vi "slow_control_2_07.vi"() -> ()   [LabVIEW 2018]
uses:
  <instrlib>/Lake Shore 335/Lake Shore 335.lvlib
  <instrlib>/CAEN PSM/CAEN PSM.lvlib
  <vilib>/DAQmx/read.llb/DAQmx Read (Analog 1D DBL NChan 1Samp).vi
  <resource>/objmgr/daqmx.rc
  ffb0d1b3-ef19-4e2e-b36e-7277177ef4b3.vi
  9a1acc8a-69db-4048-9e4c-bb07d66d2422.vi
  499f9cf5-7b15-41ea-951a-8da9be12721d.vi
  fa57f61f-0bb9-49ac-92eb-fcb40add4dbb.vi
  <vilib>/DAQmx/create/channels.llb/DAQmx Create Channel (AI-Temperature-RTD).vi
  <vilib>/DAQmx/create/channels.llb/DAQmx Create Channel (AI-Current-Basic).vi
  <vilib>/DAQmx/create/channels.llb/DAQmx Create Channel (AI-Voltage-Basic).vi
panel:
  out "Array 4":i32[](array[numeric])
  out "Array 3":i32[](array[numeric])
  out "Array 2":i32[](array[numeric])
  out "Timestamp last measured":timestamp
  out "Auto-clear":bool
  in  "Auto-clear data?":bool
  in  "Clear data":bool
  in  "Clear data every N cycles":dbl
  in  "N samples":i32=30
  out "Average Flow (SLPM)":dbl caption="Flow (SLPM)"
  out "Channel Names":string[](array[string])
  out "Heater":dbl
  out "Coldhead":dbl
  out "Cycle number":i32
  in  "Cycles to execute":dbl=5.0 format="%#_13g"
  out "Detector Pressure":dbl
  in  "N samples":i32=20
  in  "Allows tabs on \nfront panel":T1(tab)
  in  "Specify up to six temperature sensors inside \nthe detector, separated with a comma.\nNumbers only, single commas, no empty strings!":string="10,11,12,13,14,15"
  out "Valid example:":string="11,12, 13, 15 ,14 "
  in  "Anode ch.":enum16{"1", "2", "3", "4"}(ring)=enum."3"
  in  "CAEN unit selector":enum16{"CAEN 1", "CAEN 2"}(ring)
  in  "Multipliers":dbl[](array[numeric])=[1.0, 1.0, 1.0, 1.0, 1.0, 1.0, 1.0, 1.0]
  in  "Offsets\nsubtracted":dbl[](array[numeric])=[0.0, 0.0, 0.0, 0.0, 0.0, 0.0, 0.0, 0.0]
  in  "Channel Names (9207, ai8:15)":string[](array[string])=["i0", "i1", "i2", "i3", "i4", "i5", "i6", "i7"] caption="\"Other\""
  in  "Flow meter input:":T2(ring)=enum."v3"
  in  "Detector pressure input:":T2(ring)
  in  "Channel Names (9207, ai0:7)":string[](array[string])=["v0", "v1", "v2", "v3", "v4", "v5", "v6", "v7"] caption="\"Other\""
  in  "Multipliers":dbl[](array[numeric])=[0.2, 1.0, 1.0, 28.409091, 1.0, 1.0, 1.0, 1.0]
  in  "Offsets\nsubtracted":dbl[](array[numeric])=[0.002, 0.0, 0.0, 0.44376, 0.0, 0.0, 0.0, 0.0]
  in  "Voltage channels":tag[](array[tag])=["9207/ai0", "9207/ai1", "9207/ai2", "9207/ai3", "9207/ai4", "9207/ai5", "9207/ai6", "9207/ai7"]
  in  "COM-port CAEN 1":refnum<visa-resource-name>
  in  "COM-port CAEN 2":refnum<visa-resource-name>
  out "Temp B":dbl
  out "Temp A":dbl
  out "LakeShore readings 2":dbl[](array[numeric])
  in  "Run lakeshore?":bool
  in  "ID Query":bool=TRUE
  in  "COM-port LakeShore":refnum<visa-resource-name>
  in  "PID settings":cluster{"P":dbl, "I":dbl, "D":dbl}={"P"=50.0, "I"=20.0, "D"=120.0}
  in  "Setpoint (°C)":dbl=-100.0 format="%.1f"
  in  "Heater range":u16(ring) items=["Off", "Low (On)", "Medium", "High"]
  in  "Current channels":tag[](array[tag])=["9207/ai8", "9207/ai9", "9207/ai10", "9207/ai11", "9207/ai12", "9207/ai13", "9207/ai14", "9207/ai15"]
  in  "Channel Names (CAEN)":string[](array[string])=["PMT 1", "PMT 2", "Anode", "Cathode", "Top gate", "Bottom gate", "Other 1", "Other 2"]
  in  "RTD Type":i32(ring)=12481 items=["Pt3750"=12481, "Pt3851"=10071, "Pt3911"=12482, "Pt3916"=10069, "Pt3920"=10053, "Pt3928"=12483, "Custom"=10137]
  in  "Module 1 channels (slot 1)":tag[](array[tag])
  in  "Current Excitation Source":i32(ring)=10200 items=["Internal"=10200, "External"=10167, "None"=10230]
  in  "Resistance Configuration":i32(ring)=3 items=["2-Wire"=2, "3-Wire"=3, "4-Wire"=4]
  in  "R (T = 0°C):":dbl
  in  "B":dbl
  in  "A":dbl
  in  "C":dbl
  in  "Module 2 channels (slot 2)":tag[](array[tag])
  out "Det. T.":i32[](array[numeric])
  out "9207 (V; A) Converted":dbl[](array[numeric])
  out "9216 #1 (°C)":dbl[](array[numeric])
  out "9216 #2 (°C)":dbl[](array[numeric])
  out "Readouts (V, mA)":dbl[](array[numeric]) format="%0.2f"
  out "Det.P input #":i32
  out "Flow input #":i32
  in  "Repeat Alarm SMS\nevery N minutes":dbl=15.0
  in  "Test alarm":bool
  in  "Shut off heating if Alarm is active":bool
  out "Warning":bool
  in  "UPS":bool
  in  "UPS Voltage Threshold":dbl=220.0
  out "String 6":string
  out "String 5":string
  out "String 4":string
  out "String 3":string
  out "String 2":string
  out "String":string
  out "NI mod 2&3 status":bool
  in  "NI mod 2&3":bool
  in  "NI mod 1":bool
  in  "CAEN 2":bool
  in  "CAEN 1":bool
  in  "LakeShore":bool
  out "Det. P. warning":bool
  out "Boolean 6":bool
  out "Boolean 5":bool
  out "Boolean 4":bool
  out "Boolean 3":bool
  out "Boolean 2":bool
  out "Boolean":bool
  in  "T 6":bool
  in  "T 5":bool
  in  "T 4":bool
  in  "T 3":bool
  in  "T 2":bool
  in  "T 1":bool
  in  "Detector P":bool
  in  "Overpressure threshold":dbl
  in  "Underpressure threshold":dbl
  out "Comm. status":bool
  in  "High Temp threshold":dbl format="%#_13g"
  in  "Low Temp threshold":dbl format="%#_13g"
  in  "Ignore Initialization Errors":bool=TRUE caption="Ignore init. errors?"
  out "LakeShore status":bool
  out "NI mod1 (P) status":bool
  out "CAEN 1 status":bool
  out "CAEN 2 status":bool
  out "Initialization status":bool
  out "Minimum input voltage measured":dbl
  out "9207 (ai8:15, Amperes)":cluster{timestamp[], dbl[]}[](graph)
  in  "Temperature channel selector":u16(ring)=10 items=["11"=11, "12"=12, "13"=13, "14"=14, "15"=15, "16"=16, "17"=17, "Average"=666]
  out "Heater power (%)":cluster{timestamp[], dbl[]}[](graph)
  out "Flow (SLPM)":cluster{timestamp[], dbl[]}[](graph)
  out "9207 (ai0:7, Volts)":cluster{timestamp[], dbl[]}[](graph)
  out "Phase Diagram":cluster{"X":dbl, "Y":dbl}[](graph)
  out "Temperature":cluster{timestamp[], dbl[]}[](graph)
  in  "Pause?":bool
  out "Integrated Flow (SL)":dbl
  in  "Reset?":bool
  out "LakeShore readings":dbl[](array[numeric])
  in  "Temperature Channel Selector":u16(ring) items=["11"=11, "12"=12, "13"=13, "14"=14, "15"=15, "16"=16, "17"=17]
  out "Historical Large Phase Diagram":cluster{dbl[], dbl[]}[](graph)
  out "Large Phase Diagram":cluster{"X":dbl, "Y":dbl}[](graph)
  in  "Temperature Channel Selector":u16(ring)=666 items=["11"=11, "12"=12, "13"=13, "14"=14, "15"=15, "16"=16, "17"=17, "Average"=666]
  in  "Scale.Range:Minimum 8":dbl
  in  "Scale.Range:Maximum 8":dbl=4000.0
  in  "Scale.Range:Minimum 7":dbl
  in  "Scale.Range:Maximum 7":dbl=4000.0
  in  "Scale.Range:Minimum 6":dbl=-3000.0
  in  "Scale.Range:Maximum 6":dbl
  in  "Scale.Range:Minimum 5":dbl
  in  "Scale.Range:Maximum 5":dbl=3000.0
  in  "Scale.Range:Minimum 4":dbl=-5000.0
  in  "Scale.Range:Maximum 4":dbl
  in  "Scale.Range:Maximum 3":dbl=4000.0
  in  "Scale.Range:Minimum 3":dbl
  in  "Scale.Range:Maximum 2":dbl=1000.0
  in  "Scale.Range:Minimum 2":dbl
  out "CAEN 1.1":dbl(knob) scale=0.0..1000.0
  out "CAEN 1.1":string
  in  "Scale.Range:Maximum":dbl=1000.0
  in  "Scale.Range:Minimum":dbl
  out "CAEN 2.3 2":string
  out "CAEN 2.2 2":string
  out "Channel Names":string[](array[string])
  out "CAEN 2.3":dbl(knob) scale=0.0..4000.0
  out "CAEN 2.2":dbl(knob) scale=0.0..4000.0
  out "CAEN 2.1":string
  out "CAEN 2.0":string
  out "CAEN 1.3":string
  out "CAEN 1.2":string
  out "CAEN 1.0":string
  out "Channel Names":string[](array[string])
  in  "Set to zero":bool
  out "CAEN 2.1":dbl(knob)
  out "CAEN 2.0":dbl(knob) scale=0.0..3000.0
  in  "Apply Voltage":bool
  in  "VSet (V)":dbl[](array[numeric])
  in  "IMax (uA)":dbl[](array[numeric])
  in  "VMax (V)":dbl[](array[numeric])
  out "CAEN 1.3":dbl(knob)
  out "CAEN 1.2":dbl(knob) scale=0.0..4000.0
  out "CAEN 1.0":dbl(knob) scale=0.0..1000.0
  out "Vmon (V)":dbl[](array[numeric])
  out "IMon (uA)":dbl[](array[numeric])
  in  "Read V every N cycles":i16=120
  in  "Reset anode":bool
  in  "Kill every Y minutes":i32=10
  in  "Keep off for X seconds":i32=10
  out "?":bool
  out "Killed":bool
  out "Restarted":bool
  out "Anode times":dbl[](array[numeric]) format="%_12f"
  out "Anode times 2":timestamp[](array[timestamp])
  in  "Kill voltage":bool
  in  "stop":bool
  out "Voltages":dbl[](array[numeric])
  out "Started up?":bool
  out "TOBA appended":dbl[][](array[numeric])
  in  "Read T every N cycles":i32=2
  out "Time until next cycle":dbl format="%.3g"
  in  "Time per cycle (s)":i32=2 caption="Time Target (s)"
  # "<- Proof of concept for New/Old T + New P"
  # "Moving averages"
  # "NI 9216 Temperature settings"
  # "CAEN settings"
  # "NI 9207 Voltage settings"
  # "If RTD type is custom,\nspecify the Callendar-\nVan Dusen parameters"
  # "Anode connected to:"
  # "Channel:"
  # "Lakeshore settings"
  # "NI 9207 Current settings"
  # "Connection settings"
  # "Gain (P) (XX.X)"
  # "Reset (I) (XX.X)"
  # "Rate (D) (X.X%)"
  # "Move to Quick Temp tab ^"
  # "Thresholds"
  # "Alarm indicators and arms"
  # "Alarm conditions"
  # "Data"
  # "Time of last reset"
  # "Scale:"
  # "to"
  # "to"
  # "Scale:"
  # "Time of last reactivation"
  # "Settings"
  # "to"
  # "Scale:"
  # "to"
  # "Scale:"
  # "Scale:"
  # "to"
  # "Scale:"
  # "to"
  # "Scale:"
  # "to"
  # "to"
  # "Scale:"
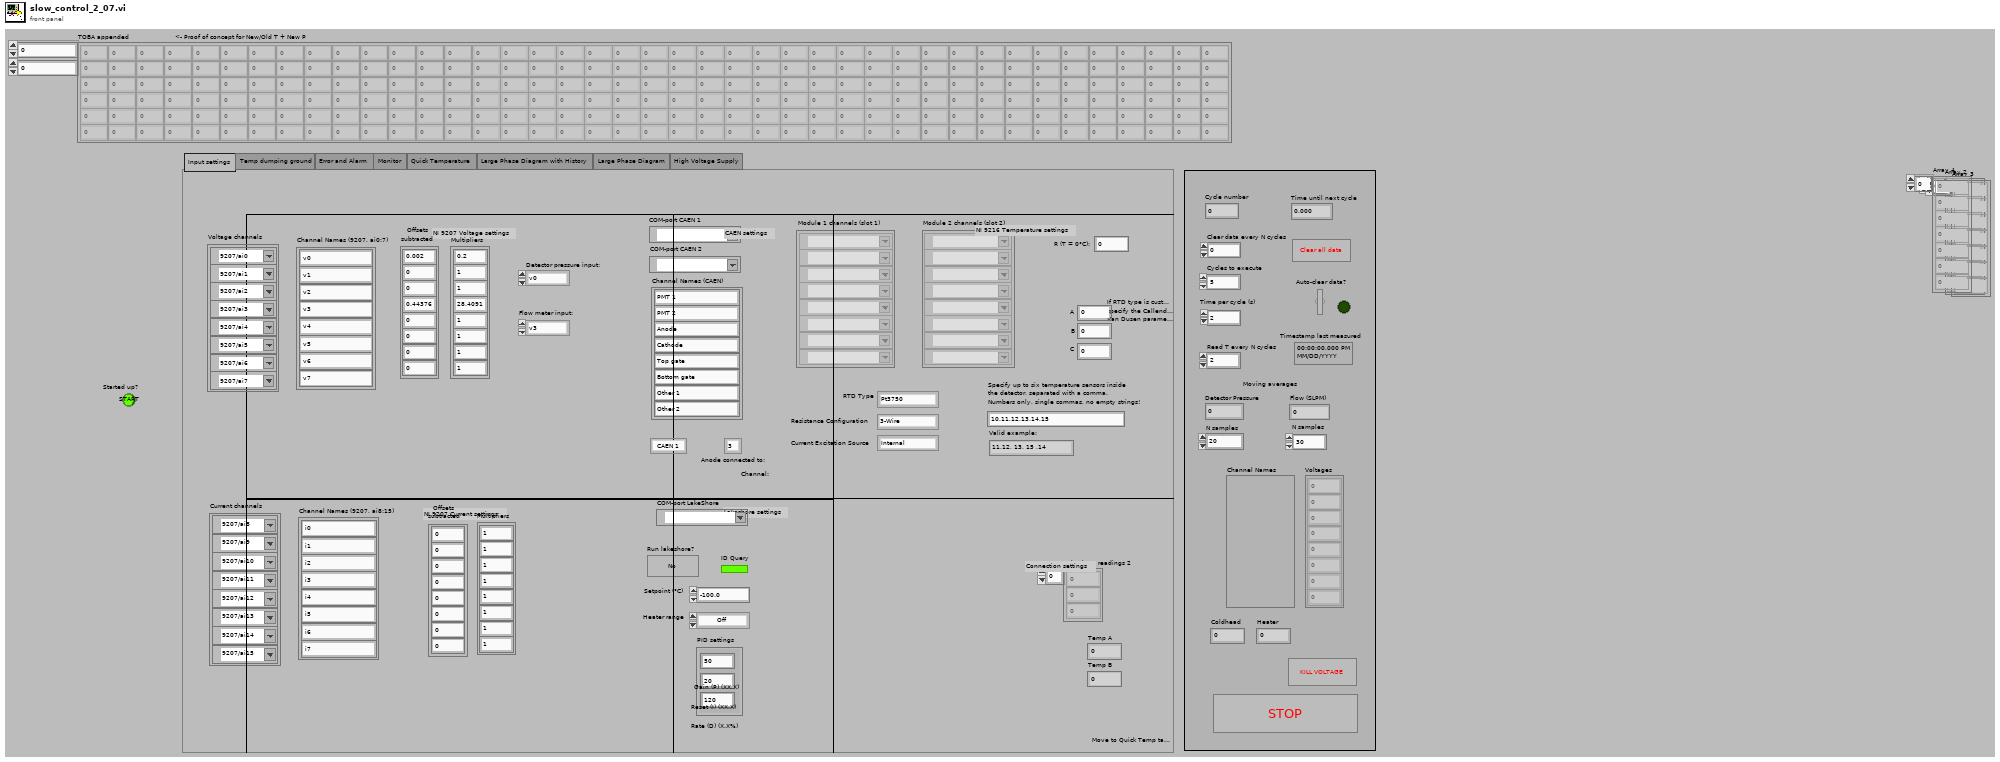
[diagram p1: front panel]
types:
  T1 = enum32{"Input settings", "Temp dumping ground", "Error and Alarm", "Monitor", "Quick Temperature", "Large Phase Diagram with History", "Large Phase Diagram", "High Voltage Supply"}
  T2 = enum16{"v0", "v1", "v2", "v3", "v4", "v5", "v6", "v7"}
  T3 = cluster{"Baud Rate":u32, "Parity":u16, "Data Bits":u16, "Stop Bits":u16, "Flow Control":u16}
  T4 = cluster{"VISA resource name out":refnum<visa-resource-name>, "error out":errorcluster}
  T5 = cluster{"task out":refnum<k21>, "error out":errorcluster}
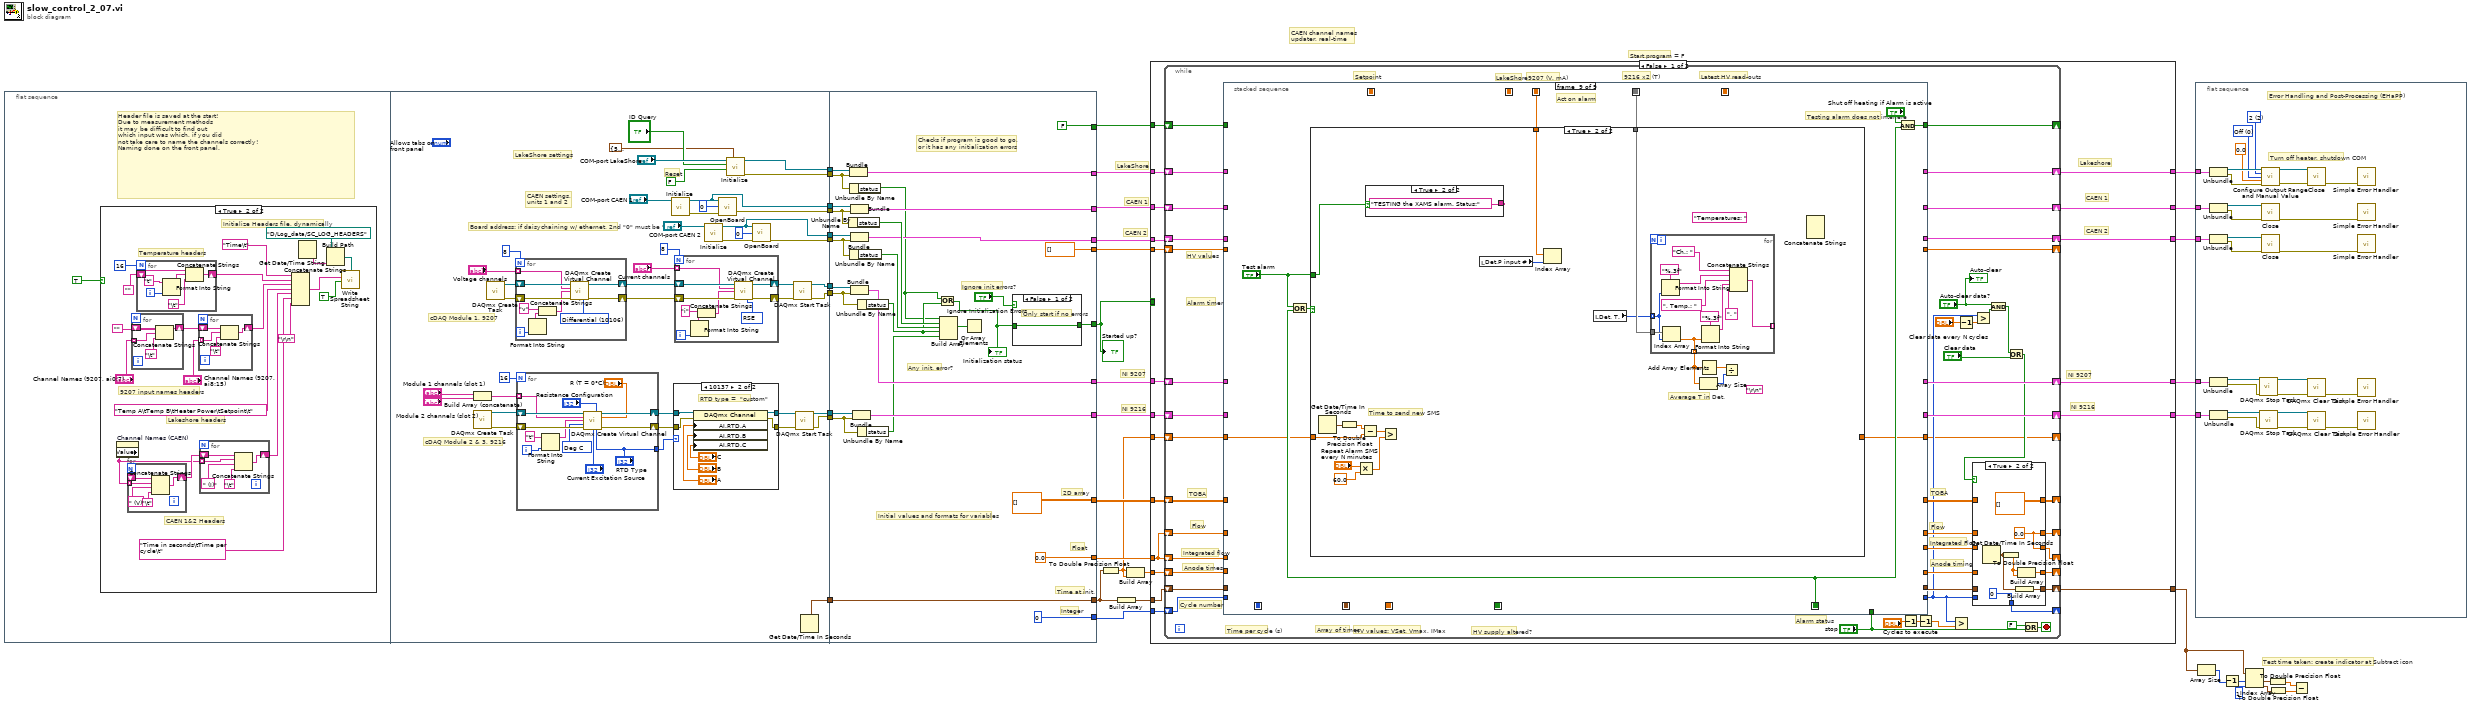
[diagram p0: block diagram]
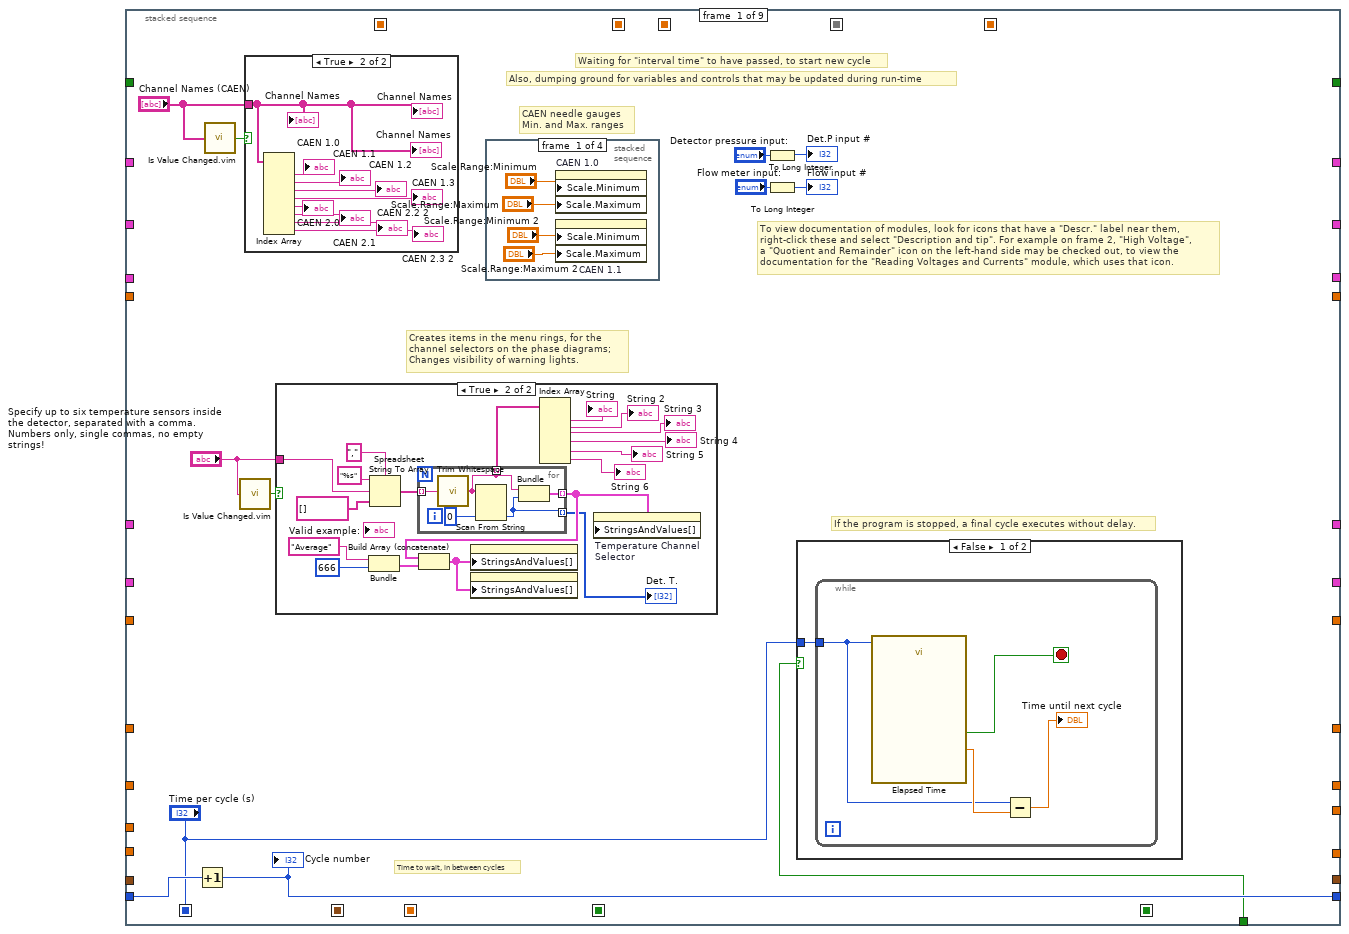
[diagram p3: hidden frame]
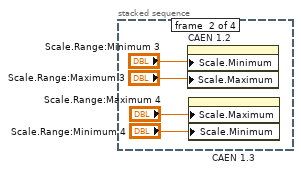
[diagram p6: hidden frame]
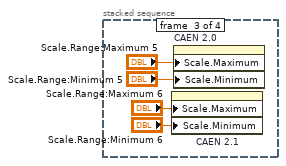
[diagram p7: hidden frame]
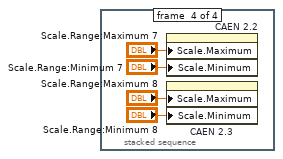
[diagram p8: hidden frame]
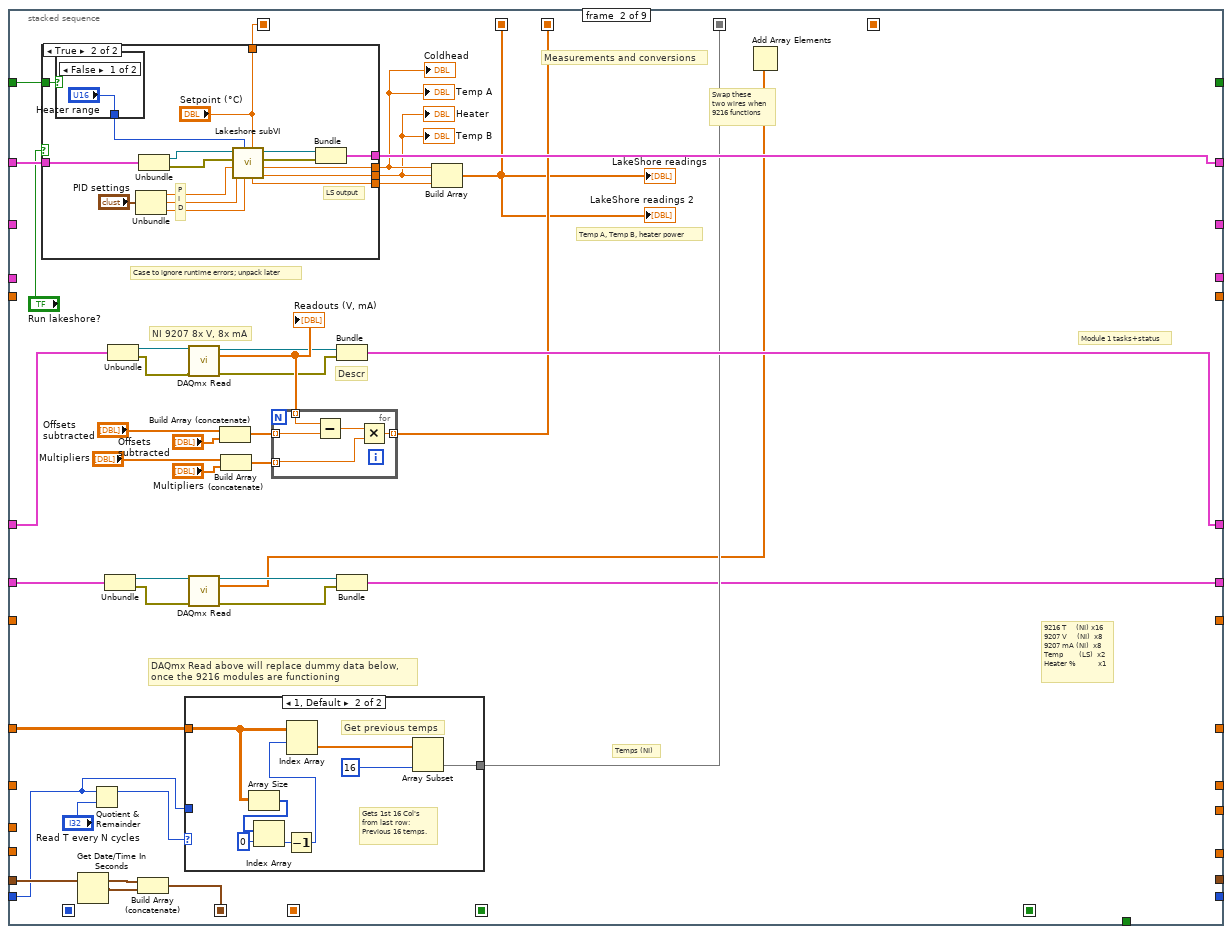
[diagram p10: hidden frame]
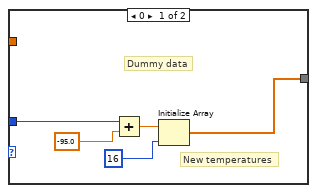
[diagram p11: hidden frame]
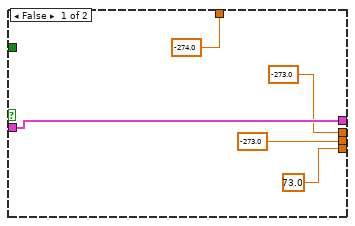
[diagram p12: hidden frame]
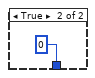
[diagram p13: hidden frame]
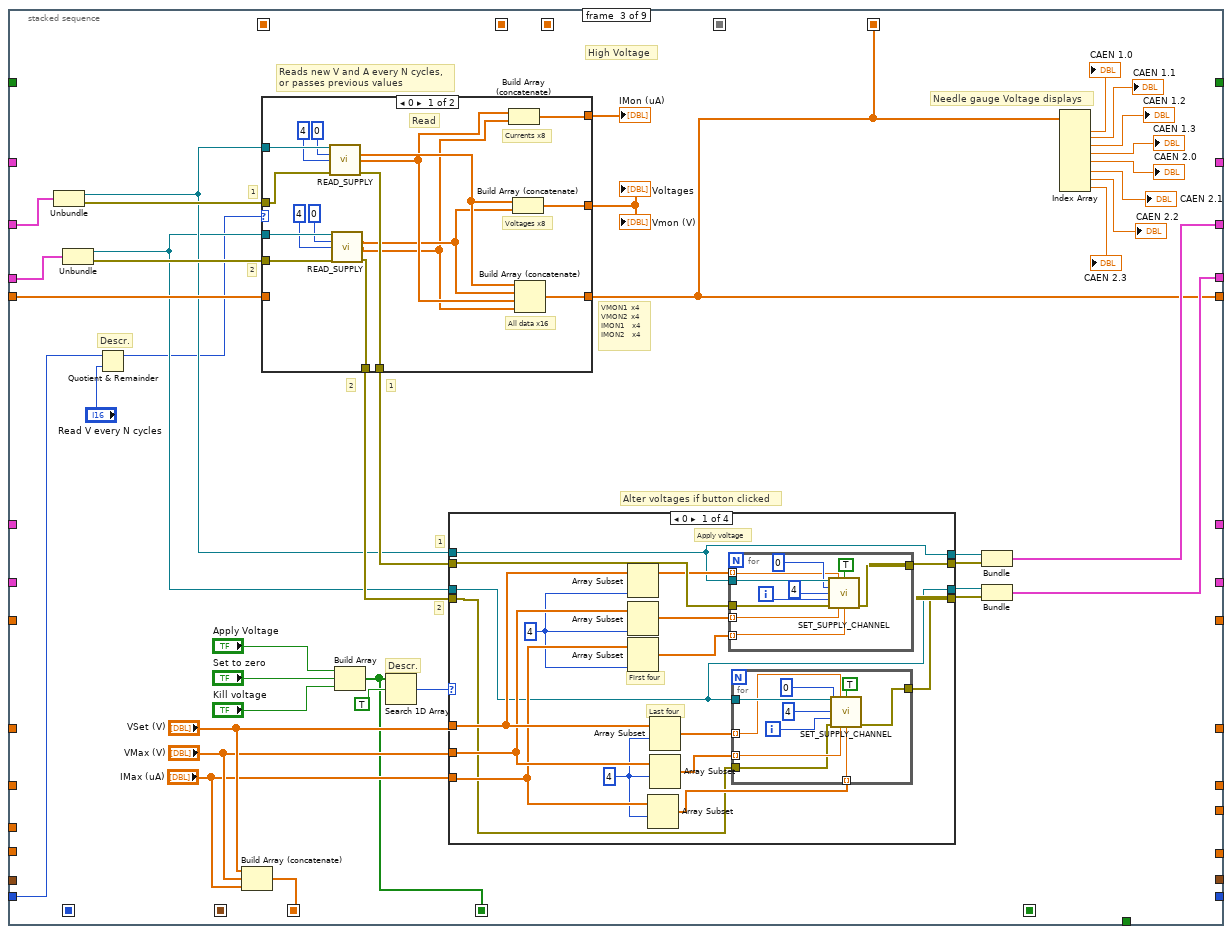
[diagram p14: hidden frame]
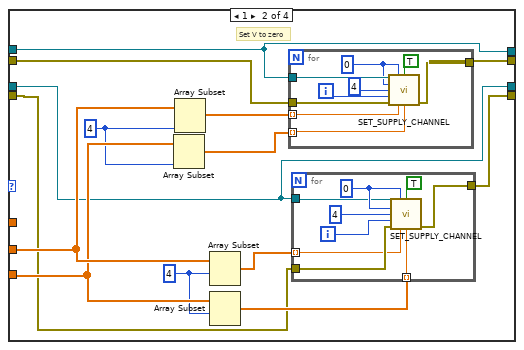
[diagram p15: hidden frame]
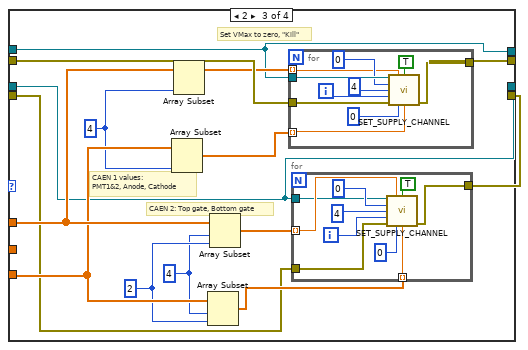
[diagram p16: hidden frame]
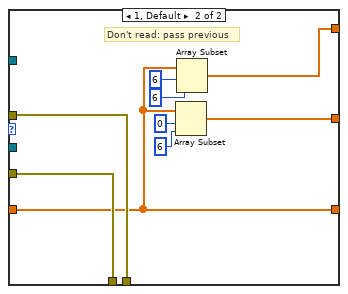
[diagram p18: hidden frame]
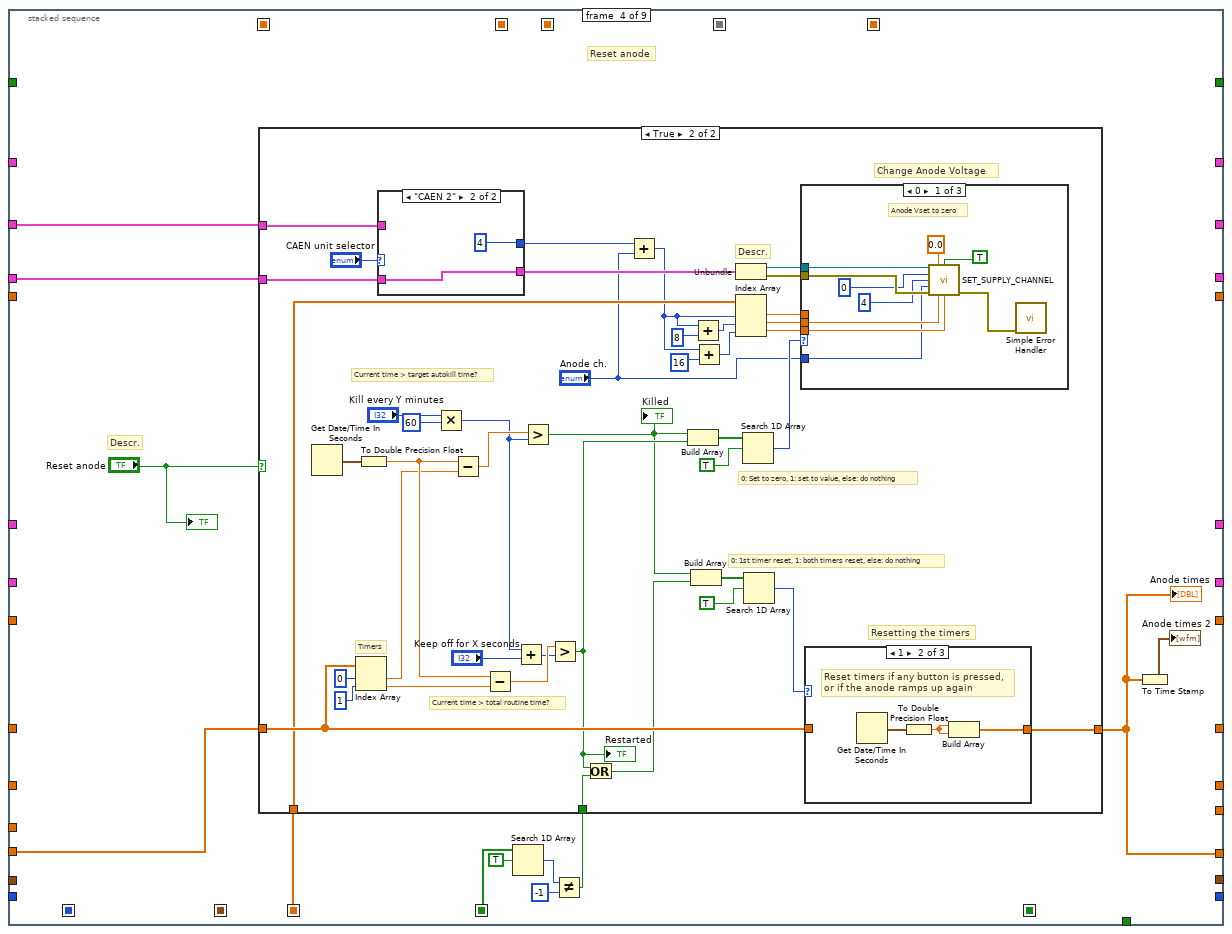
[diagram p19: hidden frame]
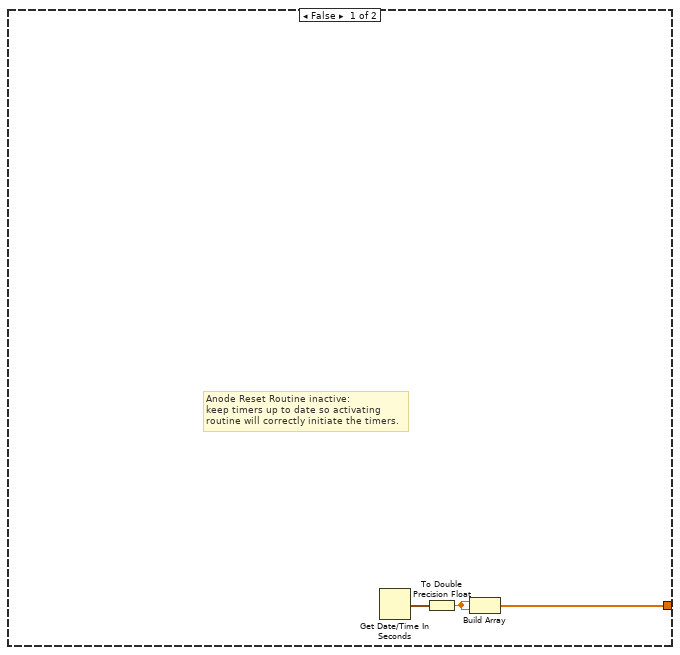
[diagram p20: hidden frame]
diagram:
  # "CAEN channel names\nupdater, real-time"
  # "NI 9216"
  # "Test time taken: create indicator at Subtract icon"
  # "NI 9207"
  # "Start program = F"
  # "CAEN 2"
  # "CAEN 1"
  # "LakeShore"
  n1 = flat-sequence {
    tunnel: [w123] -> w39
    tunnel: [w122] -> w38
    tunnel: [w110] -> w37
    tunnel: [w119] -> w36
    tunnel: [w100] -> w35
    tunnel: [w118] -> w30
    tunnel: [w114] -> w22
    tunnel: [w113] -> w21
    tunnel: [w101] -> w13
    tunnel: [w95] -> w5
    tunnel: [w94] -> w4
    tunnel: w39 -> [w195]
    tunnel: w38 -> [w194]
    tunnel: w37 -> [w192]
    tunnel: w36 -> [w191]
    tunnel: w35 -> [w181]
    tunnel: [w196] -> w19
    tunnel: [0.0] -> w18
    tunnel: [dbl[] []] -> w34
    tunnel: [dbl[][] []] -> w6
    tunnel: [0] -> w33
    tunnel: [w193] -> w32
    tunnel: [w190] -> w31
    tunnel: [w189] -> w17
    tunnel: w30 -> [w189]
    tunnel: w22 -> [w187]
    tunnel: w21 -> [w186]
    tunnel: [w185] -> w20
    tunnel: [FALSE] -> w14
    tunnel: w13 -> [w182]
    tunnel: [w180] -> w12
    tunnel: w5 -> [w172]
    tunnel: w4 -> [w171]
    tunnel: [w170] -> w3
    frame #0 {
      # "Header file is saved at the start!\nDue to measurement methods\nit may be difficult to find out\nwhich input was which, if you did\nnot take care to name the channels correctly!\nNaming done on the front panel."
      n2 = case shown="True" TRUE {
        frame False {
        }
        frame True {
          # "CAEN 1&2 Headers"
          # "Lakeshore headers"
          # "9207 input names headers"
          # "Temperature headers"
          # "Initialize Headers file, dynamically"
          n3 = property on="Channel Names (CAEN)" class="Arr (strict)"() -> ("Value"=w45:string[])  [unwired: 2 in, 2 out]
          n4 = for {
            tunnel: w45 -> [w69] mode=indexing
            shift-right: [w67] -> w46
            shift-left: _ -> [w66]
            n5 = Concatenate Strings(w66, w69, " (V)", "\t") -> (w67:string)
          }
          n6 = for {
            shift-right: [w77] -> w49
            shift-left: "" -> [w78]
            tunnel: "Channel Names (9207, ai0:7)" -> [w75] mode=indexing
            n7 = Concatenate Strings(w78, w75, "\t") -> (w77:string)
          }
          n8 = for {
            N: 16 -> [_]
            shift-right: [w79] -> w52
            shift-left: "" -> [w80]
            i -> [w84]
            n9 = Format Into String(initial string="t", w84) -> (resulting string=w82:string)  [unwired: 2 in, 1 out]
            n10 = Concatenate Strings(w80, w82, "\t") -> (w79:string)
          }
          n11 = for {
            shift-right: [w72] -> w48
            shift-left: w49 -> [w74]
            tunnel: "Channel Names (9207, ai8:15)" -> [w71] mode=indexing
            n12 = Concatenate Strings(w74, w71, "\t") -> (w72:string)
          }
          n13 = for {
            shift-right: [w62] -> w44
            shift-left: w46 -> [w63]
            tunnel: w45 -> [w61] mode=indexing
            n14 = Concatenate Strings(w63, w61, " (I)", "\t") -> (w62:string)
          }
          n15 = Concatenate Strings("Time\t", w52, w48, "Temp A\tTemp B\tHeater Power\tSetpoint\t", w44, "Time in seconds\tTime per cycle\t", "\r\n") -> (w51:string)
          n16 = Get Date/Time String() -> (date string=w55:string)  [unwired: 3 in, 1 out]
          n17 = Build Path(base path=path "D:/Log_data/SC_LOG_HEADERS" ("file path (dialog if empty)"), name or relative path=w55) -> (appended path=w56:path)
          n18 = call <vilib>:"Write Spreadsheet String.vi"("append to file? (new file:F)"=TRUE, "spreadsheet string"=w51, "file path (dialog if empty)"=w56) -> ()  [unwired: 7 in, 2 out]
        }
      }
    }
    frame #1 {
      # "cDAQ Module 2 & 3, 9216"
      # "cDAQ Module 1, 9207"
      # "Board address: if daisychaining w/ ethernet, 2nd \"0\" must be \"1\""
      # "CAEN settings,\nunits 1 and 2"
      # "Reset"
      # "LakeShore settings"
      n19 = call <vilib>:"DAQmx Create Task.vi"() -> ("task out"=w93:refnum<k21>, "error out"=w96:errorcluster)  [unwired: 14 in]
      n20 = Build Array (concatenate)("Module 1 channels (slot 1)", "Module 2 channels (slot 2)") -> (w90:tag[])
      n21 = call <vilib>:"DAQmx Create Task.vi"() -> ("task out"=w109:refnum<k21>, "error out"=w108:errorcluster)  [unwired: 14 in]
      n22 = for {
        N: 8 -> [_]
        shift-right: [w164] -> w105
        shift-left: w109 -> [w163]
        shift-right: [w165] -> w104
        shift-left: w108 -> [w161]
        tunnel: "Voltage channels" -> [w162] mode=indexing
        i -> [w167]
        w159 = 10106 items=["Default"=-1, "RSE"=10083, "NRSE"=10078, "Differential"=10106, "Pseudodifferential"=12529] ("input terminal configuration")
        n23 = Format Into String(w167) -> (resulting string=w166:string)  [unwired: 3 in, 1 out]
        n24 = Concatenate Strings("v" ("string"), w166) -> (w160:string)
        n25 = call-poly <vilib>:"DAQmx Create Virtual Channel.vi"("task in"=w163, "input terminal configuration"=w159, "physical channels"=w162, "name to assign"=w160, "error in"=w161) -> ("task out"=w164:refnum<k21>, "error out"=w165:errorcluster)  [unwired: 9 in]
      }
      n26 = for {
        N: 16 -> [_]
        shift-right: [w145] -> w89
        shift-left: w93 -> [w148]
        shift-right: [w146] -> w88
        shift-left: w96 -> [w147]
        tunnel: w90 -> [w144] mode=indexing
        tunnel: ["RTD Type"] -> w85
        i -> [w142]
        w139 = 10143 items=["Deg C"=10143, "Deg F"=10144, "Kelvins"=10325, "Deg R"=10145, "From Custom Scale"=10065] ("units")
        n27 = Format Into String(initial string="t", w142) -> (resulting string=w141:string)  [unwired: 2 in, 1 out]
        n28 = call-poly <vilib>:"DAQmx Create Virtual Channel.vi"("task in"=w148, "resistance configuration"="Resistance Configuration", "physical channels"=w144, "r0"="R (T = 0°C):", "name to assign"=w141, "units"=w139, "error in"=w147, "current excitation source"="Current Excitation Source", "rtd type"="RTD Type") -> ("task out"=w145:refnum<k21>, "error out"=w146:errorcluster)  [unwired: 5 in]
      }
      n29 = call <instrlib>:"Initialize.vi"("VISA resource name"="COM-port CAEN 1") -> ("error out"=w120:errorcluster, "VISA resource name out"=w110:refnum<visa-resource-name>)  [unwired: 9 in]
      n30 = case shown="10137" w85 {
        tunnel: w89 -> [w128 w132]
        tunnel: w88 -> [w127 w131]
        tunnel: [w128 w130] -> w87
        tunnel: [w127 w129] -> w86
        frame 0, Default {
          # "Don't need to specify the A, B, C\nvalues if RTD type is not \"custom\""
        }
        frame 10137 {
          # "RTD type =  \"custom\""
          n31 = property class="DAQmx Channel"(reference=w132, error in=w131, "AI.RTD.A"="A", "AI.RTD.B"="B", "AI.RTD.C"="C") -> (reference out=w130:refnum<k21>, error out=w129:errorcluster)
        }
      }
      n32 = for {
        N: 8 -> [_]
        shift-right: [w150] -> w102
        shift-left: w105 -> [w157]
        shift-right: [w149] -> w103
        shift-left: w104 -> [w156]
        tunnel: "Current channels" -> [w155] mode=indexing
        i -> [w154]
        w158 = 10083 items=["default"=-1, "RSE"=10083, "NRSE"=10078, "Differential"=10106, "Pseudodifferential"=12529] ("input terminal configuration")
        n33 = Format Into String(w154) -> (resulting string=w152:string)  [unwired: 3 in, 1 out]
        n34 = Concatenate Strings("i", w152) -> (w151:string)
        n35 = call-poly <vilib>:"DAQmx Create Virtual Channel.vi"("task in"=w157, "input terminal configuration"=w158, "physical channels"=w155, "name to assign"=w151, "error in"=w156) -> ("task out"=w150:refnum<k21>, "error out"=w149:errorcluster)  [unwired: 9 in]
      }
      n36 = call <instrlib>:"Initialize.vi"("VISA resource name"="COM-port CAEN 2") -> ("error out"=w115:errorcluster, "VISA resource name out"=w114:refnum<visa-resource-name>)  [unwired: 9 in]
      n37 = call <instrlib>:"OpenBoard.vi"("error in (no error)"=w120, "Board Address"=0, "VISA resource name"=w110) -> ("error out"=w119:errorcluster)  [unwired: 7 in, 1 out]
      n38 = call <instrlib>:"Initialize.vi"("Serial Configuration"=T3 {"Baud Rate"=57600, "Parity"=1, "Data Bits"=7, "Stop Bits"=10, "Flow Control"=0}, "Reset (True)"=FALSE ("Reset (LakeShore)"), "ID Query (True)"="ID Query", "VISA resource name"="COM-port LakeShore") -> ("error out"=w122:errorcluster, "VISA resource name out"=w123:refnum<visa-resource-name>)  [unwired: 6 in]
      n39 = call <instrlib>:"OpenBoard.vi"("error in (no error)"=w115, "Board Address"=u8 0, "VISA resource name"=w114) -> ("error out"=w113:errorcluster)  [unwired: 7 in, 1 out]
      n40 = call <vilib>:"DAQmx Start Task.vi"("task/channels in"=w102, "error in"=w103) -> ("task out"=w101:refnum<k21>, "error out"=w100:errorcluster)  [unwired: 12 in]
      n41 = call <vilib>:"DAQmx Start Task.vi"("task/channels in"=w87, "error in"=w86) -> ("task out"=w95:refnum<k21>, "error out"=w94:errorcluster)  [unwired: 12 in]
      n42 = Get Date/Time In Seconds() -> (seconds since 1Jan1904=w118:timestamp)
    }
    frame #2 {
      # "Initial values and formats for variables"
      # "Time at init."
      # "Integer"
      # "2D array"
      # "Float"
      # "Checks if program is good to go,\nor it has any initialization errors"
      # "Ignore init errors?"
      # "Any init. error?"
      n43 = Unbundle By Name(w191) -> ("status"=w197:bool)
      n44 = Unbundle By Name(w194) -> ("status"=w174:bool)
      n45 = Bundle("VISA resource name out"=w195, "error out"=w194) -> (w193:T4)  [unwired: 1 in]
      n46 = Unbundle By Name(w186) -> ("status"=w188:bool)
      n47 = Bundle("VISA resource name out"=w187, "error out"=w186) -> (w185:T4)  [unwired: 1 in]
      n48 = Bundle("task out"=w182, "error out"=w181) -> (w180:T5)  [unwired: 1 in]
      n49 = Bundle("VISA resource name out"=w192, "error out"=w191) -> (w190:T4)  [unwired: 1 in]
      n50 = Bundle("task out"=w172, "error out"=w171) -> (w170:T5)  [unwired: 1 in]
      n51 = Unbundle By Name(w181) -> ("status"=w175:bool)
      n52 = Unbundle By Name(w171) -> ("status"=w169:bool)
      n53 = Or(x=w174, y=w175) -> (x .or. y?=w173:bool)
      "Initialization status" <- w173
      n54 = Build Array(w174, w197, w175, w188, w169) -> (w198:bool[])
      n55 = Or Array Elements(Boolean array=w198) -> ()  [unwired: 1 out]
      n56 = case shown="False" "Ignore Initialization Errors" {
        tunnel: [w199 FALSE] -> w196
        tunnel: w173 -> [w199 _]
        frame False {
          # "Only start if no errors"
        }
        frame True {
          # "Always start program"
        }
      }
    }
  }
  n57 = To Double Precision Float(number=w17) -> (double precision float=w1:dbl)
  n58 = Build Array(w17) -> (w29:timestamp[])
  n59 = Build Array(w1, w1) -> (w16:dbl[])
  n60 = case shown="False" w19 {
    selector: w19 -> [_ w951]
    tunnel: [_ w951] -> _
    tunnel: w34 -> [w212 _]
    tunnel: w33 -> [w219 _]
    tunnel: w6 -> [w218 _]
    tunnel: w32 -> [w213 w949]
    tunnel: w31 -> [w215 w948]
    tunnel: w29 -> [w217 _]
    tunnel: [w216 timestamp[] []] -> w25
    tunnel: w20 -> [w214 w947]
    tunnel: w18 -> [w208 _]
    tunnel: w16 -> [w211 _]
    tunnel: [w210 w949] -> w15
    tunnel: w14 -> [w209 _]
    tunnel: w12 -> [w207 w946]
    tunnel: [w206 w948] -> w11
    tunnel: [w205 w947] -> w10
    tunnel: [w204 w946] -> w9
    tunnel: w3 -> [w203 w945]
    tunnel: [w202 w945] -> w2
    tunnel: w1 -> [w201 _]
    frame False {
      # "NI 9216"
      # "NI 9207"
      # "CAEN 2"
      # "CAEN 1"
      # "Lakeshore"
      n61 = while {
        shift-right: [w228] -> _
        shift-left: w219 -> [w266]
        shift-right: [w241] -> _
        shift-left: w218 -> [w255]
        shift-right: [w233] -> w216
        shift-left: w217 -> [w263]
        shift-right: [w257] -> w206
        shift-left: w215 -> [w250]
        shift-right: [w259] -> _
        shift-left: w212 -> [w262]
        shift-right: [w256] -> w205
        shift-left: w214 -> [w261]
        shift-right: [w258] -> w210
        shift-left: w213 -> [w260]
        shift-right: [w237] -> _
        shift-left: w208 -> [w252]
        shift-right: [w239] -> _
        shift-left: w208 -> [w253]
        shift-right: [w235] -> _
        shift-left: w211 -> [w251]
        shift-right: [w222] -> _
        shift-left: w209 -> [w249]
        shift-right: [w247] -> w204
        shift-left: w207 -> [w248]
        shift-right: [w245] -> w202
        shift-left: w203 -> [w246]
        shift-right: [w220] -> _
        shift-left: w201 -> [w221]
        stop <- w264 stop-if-true
        # "Alarm timer"
        # "Alarm status"
        # "LakeShore"
        # "9216 x2 (T)"
        # "9207 (V, mA)"
        # "HV supply altered?"
        # "Setpoint"
        # "Anode timing"
        # "Anode times"
        # "Integrated flow"
        # "Flow"
        # "Flow"
        # "Integrated Flow"
        # "TOBA"
        # "Array of times"
        # "Latest HV read-outs"
        # "Time per cycle (s)"
        # "Cycle number"
        # "HV values: VSet, Vmax, IMax"
        # "HV values"
        # "TOBA"
        n62 = stacked-sequence {
          seq-local: [_ _ w433 _ _ _ _ _ _] -> [_ _ _ w605 _ _ _ _ _]
          seq-local: ["Time per cycle (s)" _ _ _ _ _ _ _ _] -> [_ _ _ _ _ _ w814 _ _]
          seq-local: [_ _ w424 _ _ _ _ _ _] -> [_ _ _ _ _ _ w816 _ _]
          seq-local: [_ w377 _ _ _ _ _ _ _] -> [_ _ _ _ w696 w716 _ _ _]
          seq-local: [_ _ w427 _ _ _ _ _ _] -> [_ _ _ w608 _ _ _ _ _]
          seq-local: [_ w370 _ _ _ _ _ _ _] -> [_ _ _ _ _ _ w831 _ _]
          seq-local: [_ w365 _ _ _ _ _ _ _] -> [_ _ _ _ w691 w741 w818 w873 w910]
          seq-local: [_ w364 _ _ _ _ _ _ _] -> [_ _ _ _ w690 w732 w819 w877 w909]
          seq-local: [_ w352 _ _ _ _ _ _ _] -> [_ _ _ _ w689 w739 w817 _ _]
          seq-local: [_ _ _ _ _ _ _ w833 _] -> [_ _ _ _ _ _ _ _ w912]
          tunnel: [w290 _ _ _ _ _ _ _ _] -> w227
          tunnel: "stop" -> [w289 _ _ _ _ _ _ _ _]
          tunnel: w266 -> [w291 w366 w455 _ _ _ _ _ _]
          tunnel: w255 -> [_ w367 _ _ _ w742 _ _ _]
          tunnel: [_ _ _ _ _ w718 _ _ _] -> w242
          tunnel: w263 -> [_ w379 _ _ _ _ _ _ _]
          tunnel: w250 -> [_ _ w462 w606 _ _ _ w893 _]
          tunnel: w262 -> [_ _ w460 _ _ _ _ _ _]
          tunnel: w261 -> [_ _ w459 w597 _ _ _ w892 _]
          tunnel: w260 -> [_ w380 _ _ _ _ _ w891 _]
          tunnel: [_ w381 _ _ _ _ _ _ _] -> w258
          tunnel: [_ _ w424 _ _ _ _ _ _] -> w259
          tunnel: [_ _ w441 _ _ _ _ _ _] -> w257
          tunnel: [_ _ w438 _ _ _ _ _ _] -> w256
          tunnel: [_ _ _ _ _ w716 _ _ _] -> w234
          tunnel: w252 -> [_ _ _ _ w694 _ _ _ _]
          tunnel: w253 -> [_ _ _ _ w695 _ _ _ _]
          tunnel: w251 -> [_ _ _ w607 _ _ _ _ _]
          tunnel: [_ _ _ w601 _ _ _ _ _] -> w236
          tunnel: w249 -> [_ w373 _ _ _ _ _ _ _]
          tunnel: w248 -> [_ w372 _ _ _ _ _ w890 _]
          tunnel: [_ w368 _ _ _ _ _ _ _] -> w247
          tunnel: [_ _ _ _ w693 _ _ _ _] -> w238
          tunnel: [_ _ _ _ w692 _ _ _ _] -> w240
          tunnel: w246 -> [_ w351 _ _ _ _ _ w878 _]
          tunnel: [_ w346 _ _ _ _ _ _ _] -> w245
          tunnel: [_ _ _ _ _ _ _ _ w914] -> w222
          tunnel: w221 -> [_ _ _ _ _ _ _ _ w908]
          tunnel: [_ _ _ _ _ _ _ _ w907] -> w220
          frame #0 {
            # "Creates items in the menu rings, for the channel selectors on the phase diagrams;\nChanges visibility of warning lights."
            # "Also, dumping ground for variables and controls that may be updated during run-time"
            # "CAEN needle gauges\nMin. and Max. ranges"
            # "To view documentation of modules, look for icons that have a \"Descr.\" label near them,\nright-click these and select \"Description and tip\". For example on frame 2, \"High Voltage\",\na \"Quotient and Remainder\" icon on the left-hand side may be checked out, to view the\ndocumentation for the \"Reading Voltages and Currents\" module, which uses that icon."
            # "Time to wait, in between cycles"
            # "If the program is stopped, a final cycle executes without delay."
            # "Waiting for \"interval time\" to have passed, to start new cycle"
            n63 = Increment(x=w291) -> (x+1=w290:i32)
            "Cycle number" <- w290
            n64 = call "Is Value Changed.vim"("value"="Channel Names (CAEN)") -> ("changed or first call?"=w280:bool)
            n65 = call "Is Value Changed.vim"("value"="Specify up to six temperature sensors inside \nthe detector, separated with a comma.\nNumbers only, single commas, no empty strings!") -> ("changed or first call?"=w282:bool)
            n66 = case shown="True" w280 {
              tunnel: "Channel Names (CAEN)" -> [_ w292]
              frame False {
              }
              frame True {
                n67 = Index Array(array=w292) -> (element #1=→"CAEN 1.0":string, element #2=→"CAEN 1.1":string, element #3=→"CAEN 1.2":string, element #4=→"CAEN 1.3":string, element #5=→"CAEN 2.0":string, element #6=→"CAEN 2.1":string, element #7=→"CAEN 2.2 2":string, element #8=→"CAEN 2.3 2":string)  [unwired: 8 in]
                "Channel Names" <- w292
                "Channel Names" <- w292
                "Channel Names" <- w292
              }
            }
            n68 = case shown="True" w282 {
              tunnel: "Specify up to six temperature sensors inside \nthe detector, separated with a comma.\nNumbers only, single commas, no empty strings!" -> [_ w302]
              frame False {
              }
              frame True {
                n69 = Bundle("Average", 666) -> (w308:cluster{string, i32})  [unwired: 1 in]
                n70 = Spreadsheet String To Array(delimiter (Tab)=",", format string="%s", spreadsheet string=w302, array type (2D Dbl)=string[] []) -> (array=w311:string[])
                n71 = for {
                  tunnel: w311 -> [w323] mode=indexing
                  tunnel: [w321] -> w310 mode=indexing
                  tunnel: [w320] -> w301 mode=indexing
                  tunnel: [w319] -> w312 mode=indexing
                  n72 = call <vilib>:"Trim Whitespace.vi"("string"=w323) -> ("trimmed string"=w319:string)  [unwired: 1 in]
                  n73 = Scan From String(input string=w319, default 1=0) -> (output 1=w320:i32)  [unwired: 3 in, 3 out]
                  n74 = Bundle("trimmed string"=w319, w320) -> (w321:cluster{"trimmed string":string, i32})  [unwired: 1 in]
                }
                "Det. T." <- w301
                n75 = Build Array (concatenate)(w310, w308) -> (w309:cluster{"trimmed string":string, i32}[])
                n76 = property on="Temperature channel selector" class="Ring (strict)"("StringsAndValues[]"=w309) -> ()  [unwired: 2 in, 2 out]
                n77 = property on="Temperature Channel Selector" class="Ring (strict)"("StringsAndValues[]"=w309) -> ()  [unwired: 2 in, 2 out]
                n78 = Index Array(array=w312) -> (element #1=→"String":string, element #2=→"String 2":string, element #3=→"String 3":string, element #4=→"String 4":string, element #5=→"String 5":string, element #6=→"String 6":string)  [unwired: 6 in]
                n79 = property on="Temperature Channel Selector" class="Ring (strict)"("StringsAndValues[]"=w310) -> ()  [unwired: 2 in, 2 out]
              }
            }
            n80 = stacked-sequence {
              frame #0 {
                n81 = property on="CAEN 1.0" class="Knob (strict)"("Scale.Minimum"="Scale.Range:Minimum", "Scale.Maximum"="Scale.Range:Maximum") -> ()  [unwired: 2 in, 2 out]
                n82 = property on="CAEN 1.1" class="Knob (strict)"("Scale.Minimum"="Scale.Range:Minimum 2", "Scale.Maximum"="Scale.Range:Maximum 2") -> ()  [unwired: 2 in, 2 out]
              }
              frame #1 {
                n83 = property on="CAEN 1.2" class="Knob (strict)"("Scale.Minimum"="Scale.Range:Minimum 3", "Scale.Maximum"="Scale.Range:Maximum 3") -> ()  [unwired: 2 in, 2 out]
                n84 = property on="CAEN 1.3" class="Knob (strict)"("Scale.Maximum"="Scale.Range:Maximum 4", "Scale.Minimum"="Scale.Range:Minimum 4") -> ()  [unwired: 2 in, 2 out]
              }
              frame #2 {
                n85 = property on="CAEN 2.1" class="Knob (strict)"("Scale.Maximum"="Scale.Range:Maximum 6", "Scale.Minimum"="Scale.Range:Minimum 6") -> ()  [unwired: 2 in, 2 out]
                n86 = property on="CAEN 2.0" class="Knob (strict)"("Scale.Maximum"="Scale.Range:Maximum 5", "Scale.Minimum"="Scale.Range:Minimum 5") -> ()  [unwired: 2 in, 2 out]
              }
              frame #3 {
                n87 = property on="CAEN 2.2" class="Knob (strict)"("Scale.Maximum"="Scale.Range:Maximum 7", "Scale.Minimum"="Scale.Range:Minimum 7") -> ()  [unwired: 2 in, 2 out]
                n88 = property on="CAEN 2.3" class="Knob (strict)"("Scale.Maximum"="Scale.Range:Maximum 8", "Scale.Minimum"="Scale.Range:Minimum 8") -> ()  [unwired: 2 in, 2 out]
              }
            }
            n89 = To Long Integer(number="Detector pressure input:") -> (32bit integer=→"Det.P input #":i32)
            n90 = To Long Integer(number="Flow meter input:") -> (32bit integer=→"Flow input #":i32)
            n91 = case shown="False" w289 {
              tunnel: "Time per cycle (s)" -> [w340 _]
              frame False {
                n92 = while {
                  tunnel: w340 -> [w342]
                  stop <- w344 stop-if-true
                  n93 = call "Elapsed Time"("Time Target (s)"=w342) -> ("Elapsed Time (s)"=w343:dbl, "Time has Elapsed"=w344:bool)  [unwired: 11 in, 6 out]
                  n94 = Subtract(x=w342, y=w343) -> (x-y=→"Time until next cycle":dbl)
                }
              }
              frame True {
              }
            }
          }
          frame #1 {
            # "DAQmx Read above will replace dummy data below,\nonce the 9216 modules are functioning"
            # "Swap these\ntwo wires when\n9216 functions"
            # "Descr"
            # "NI 9207 8x V, 8x mA"
            # "Case to ignore runtime errors; unpack later"
            # "Module 1 tasks+status"
            # "Temps (NI)"
            # "9216 T     (NI) x16\n9207 V     (NI)  x8\n9207 mA (NI)  x8\nTemp        (LS)  x2\nHeater %           x1"
            # "Temp A, Temp B, heater power"
            # "Measurements and conversions"
            n95 = case shown="True" "Run lakeshore?" {
              tunnel: [w404 w412] -> w381
              tunnel: w380 -> [w404 w411]
              tunnel: [-273.0 ("Input A") w410] -> w376
              tunnel: [-273.0 ("Input B") w409] -> w375
              tunnel: [73.0 ("Heater 1 (%)") w408] -> w374
              tunnel: w373 -> [_ w407]
              tunnel: [-274.0 "Setpoint (°C)"] -> w370
              frame False {
              }
              frame True {
                # "LS output"
                # "P\nI\nD"
                n96 = case shown="False" w407 {
                  tunnel: ["Heater range" 0] -> w415
                  frame False {
                  }
                  frame True {
                  }
                }
                n97 = Unbundle("PID settings") -> ("P"=w418:dbl, "I"=w417:dbl, "D"=w416:dbl)
                n98 = Unbundle(w411) -> ("VISA resource name out"=w420:refnum<visa-resource-name>, "error out"=w419:errorcluster)
                n99 = call "Lakeshore subVI.vi"("Setpoint"="Setpoint (°C)", "Rate (D) (X.X %)"=w416, "Range"=w415, "Reset (I) (XX.X)"=w417, "Gain (P) (XX.X)"=w418, "error in (no error)"=w419, "VISA resource name"=w420) -> ("Input B"=w409:dbl, "Input A"=w410:dbl, "error out"=w413:errorcluster, "VISA resource name out"=w414:refnum<visa-resource-name>, "Heater 1 (%)"=w408:dbl)
                n100 = Bundle("VISA resource name out"=w414, "error out"=w413) -> (w412:T4)  [unwired: 1 in]
              }
            }
            "Temp A" <- w376
            "Temp B" <- w375
            "Heater" <- w375
            "Coldhead" <- w376
            n101 = Get Date/Time In Seconds() -> (seconds since 1Jan1904=w378:timestamp)
            n102 = Quotient & Remainder(x=w366, y="Read T every N cycles") -> (x-y*floor(x/y)=w369:i32)  [unwired: 1 out]
            n103 = Unbundle(w351) -> ("task out"=w350:refnum<k21>, "error out"=w349:errorcluster)
            n104 = Unbundle(w372) -> ("task out"=w356:refnum<k21>, "error out"=w355:errorcluster)
            n105 = Build Array (concatenate)(w379, w378) -> (w377:timestamp[])
            n106 = case shown="1, Default" w369 {
              tunnel: w367 -> [_ w397]
              tunnel: [w390 w393] -> w364
              tunnel: w366 -> [w389 _]
              frame 0 {
                # "Dummy data"
                # "New temperatures"
                n107 = Add(x=w389, y=-95.0 ("element")) -> (x+y=w392:dbl)
                n108 = Initialize Array(w392, 16) -> (w390:dbl[])
              }
              frame 1, Default {
                # "Gets 1st 16 Col's\nfrom last row:\nPrevious 16 temps."
                # "Get previous temps"
                n109 = Array Size(array=w397) -> (size(s)=w399:i32[])
                n110 = Index Array(array=w399, index=0) -> (element=w400:i32)
                n111 = Decrement(x=w400) -> (x-1=w396:i32)
                n112 = Index Array(array=w397, index (row)=w396) -> (element=w395:dbl[])  [unwired: 1 in]
                n113 = Array Subset(array=w395, length=16) -> (w393:dbl[])  [unwired: 1 in]
              }
            }
            n114 = call-poly <vilib>:"DAQmx Read.vi"("task/channels in"=w356, "error in"=w355) -> ("task out"=w354:refnum<k21>, "data"=w363:dbl[], "error out"=w353:errorcluster)  [unwired: 11 in]
            "Readouts (V, mA)" <- w363
            n115 = call-poly <vilib>:"DAQmx Read.vi"("task/channels in"=w350, "error in"=w349) -> ("task out"=w348:refnum<k21>, "data"=w345:dbl[], "error out"=w347:errorcluster)  [unwired: 11 in]
            n116 = Build Array (concatenate)("Offsets\nsubtracted", "Offsets\nsubtracted") -> (w357:dbl[])
            n117 = Build Array (concatenate)("Multipliers", "Multipliers") -> (w360:dbl[])
            n118 = for {
              tunnel: w357 -> [w387] mode=indexing
              tunnel: w363 -> [w386] mode=indexing
              tunnel: w360 -> [w384] mode=indexing
              tunnel: [w383] -> w365 mode=indexing
              n119 = Subtract(x=w386, y=w387) -> (x-y=w385:dbl)
              n120 = Multiply(x=w385, y=w384) -> (x*y=w383:dbl)
            }
            n121 = Bundle("task out"=w354, "error out"=w353) -> (w368:T5)  [unwired: 1 in]
            n122 = Bundle("task out"=w348, "error out"=w347) -> (w346:T5)  [unwired: 1 in]
            n123 = Build Array(w376, w375, w374) -> (w352:dbl[])
            "LakeShore readings" <- w352
            "LakeShore readings 2" <- w352
            n124 = Add Array Elements(numeric array=w345) -> ()  [unwired: 1 out]
          }
          frame #2 {
            # "Alter voltages if button clicked"
            # "2"
            # "1"
            # "Descr."
            # "Descr."
            # "VMON1  x4 \nVMON2  x4\nIMON1    x4\nIMON2    x4"
            # "Needle gauge Voltage displays"
            # "1"
            # "2"
            # "1"
            # "2"
            # "Reads new V and A every N cycles,\nor passes previous values"
            # "High Voltage"
            n125 = Unbundle(w462) -> ("VISA resource name out"=w444:refnum<visa-resource-name>, "error out"=w461:errorcluster)
            n126 = Unbundle(w459) -> ("VISA resource name out"=w443:refnum<visa-resource-name>, "error out"=w458:errorcluster)
            n127 = Quotient & Remainder(x=w455, y="Read V every N cycles") -> (x-y*floor(x/y)=w428:i32)  [unwired: 1 out]
            n128 = Build Array (concatenate)("VSet (V)", "VMax (V)", "IMax (uA)") -> (w433:dbl[])
            n129 = case shown="0" w428 {
              tunnel: w444 -> [w587 _]
              tunnel: w461 -> [w586 w595]
              tunnel: w460 -> [_ w591]
              tunnel: w443 -> [w577 _]
              tunnel: w458 -> [w574 w596]
              tunnel: [w573 w596] -> w445
              tunnel: [w583 w595] -> w446
              tunnel: [w582 w591] -> w424
              tunnel: [w580 w592] -> w457
              tunnel: [w578 w588] -> w456
              frame 0 {
                # "All data x16"
                # "Voltages x8"
                # "Currents x8"
                # "Read"
                n130 = call "READ_SUPPLY.vi"("VISA resource name"=w587, "Board address"=u8 0, "NChannels"=u8 4, "error in (no error)"=w586) -> ("VMon values (V)"=w581:dbl[], "IMon values (uA)"=w579:dbl[], "error out"=w583:errorcluster)  [unwired: 9 in]
                n131 = call "READ_SUPPLY.vi"("VISA resource name"=w577, "Board address"=u8 0, "NChannels"=u8 4, "error in (no error)"=w574) -> ("VMon values (V)"=w572:dbl[], "IMon values (uA)"=w571:dbl[], "error out"=w573:errorcluster)  [unwired: 9 in]
                n132 = Build Array (concatenate)(w579, w571) -> (w578:dbl[])
                n133 = Build Array (concatenate)(w581, w572) -> (w580:dbl[])
                n134 = Build Array (concatenate)(w581, w572, w579, w571) -> (w582:dbl[])
              }
              frame 1, Default {
                # "Don't read: pass previous"
                n135 = Array Subset(array=w591, index=0, length=6) -> (w592:dbl[])
                n136 = Array Subset(array=w591, index=6, length=6) -> (w588:dbl[])
              }
            }
            "Voltages" <- w457
            "Vmon (V)" <- w457
            "IMon (uA)" <- w456
            n137 = Build Array("Apply Voltage", "Set to zero", "Kill voltage") -> (w427:bool[])
            n138 = Search 1D Array(1D array=w427, element=TRUE) -> (index of element=w447:i32)  [unwired: 1 in]
            n139 = case shown="0" w447 {
              tunnel: w446 -> [w479 w513 w546 w567]
              tunnel: w445 -> [w466 w503 w535 w569]
              tunnel: w444 -> [w475 w510 w543 w570]
              tunnel: w443 -> [w464 w501 w533 w568]
              tunnel: [w476 w511 w544 w567] -> w437
              tunnel: [w475 w510 w543 w570] -> w442
              tunnel: [w463 w500 w532 w569] -> w439
              tunnel: [w464 w501 w533 w568] -> w440
              tunnel: "VSet (V)" -> [w473 _ w541 _]
              tunnel: "VMax (V)" -> [w472 w508 _ _]
              tunnel: "IMax (uA)" -> [w471 w507 w540 _]
              frame 0 {
                w465 = 4 ("length")
                w470 = 4 ("length")
                # "Last four"
                # "First four"
                # "Apply voltage"
                n140 = Array Subset(array=w473, length=w470) -> (w478:dbl[])  [unwired: 1 in]
                n141 = Array Subset(array=w472, length=w470) -> (w477:dbl[])  [unwired: 1 in]
                n142 = Array Subset(array=w471, length=w470) -> (w474:dbl[])  [unwired: 1 in]
                n143 = Array Subset(array=w471, index=w465) -> (w467:dbl[])  [unwired: 1 in]
                n144 = Array Subset(array=w473, index=w465) -> (w469:dbl[])  [unwired: 1 in]
                n145 = Array Subset(array=w472, index=w465) -> (w468:dbl[])  [unwired: 1 in]
                n146 = for {
                  tunnel: w475 -> [w498]
                  tunnel: w479 -> [w497]
                  tunnel: w478 -> [w494] mode=indexing
                  tunnel: w477 -> [w492] mode=indexing
                  tunnel: w474 -> [w491] mode=indexing
                  tunnel: [w490] -> w476
                  i -> [w499]
                  n147 = call "SET_SUPPLY_CHANNEL.vi"("VISA resource name"=w498, "Voltage Level (0.0 V)"=w494, "Enable (OFF)"=TRUE, "Board address"=u8 0, "NChannels"=u8 4, "Channel (0)"=w499, "error in (no error)"=w497, "Voltage Max (0.0 V)"=w492, "Current Limit (0.00 uA)"=w491) -> ("error out"=w490:errorcluster)  [unwired: 6 in]
                }
                n148 = for {
                  tunnel: w464 -> [w489]
                  tunnel: w466 -> [w483]
                  tunnel: w469 -> [w488] mode=indexing
                  tunnel: w468 -> [w487] mode=indexing
                  tunnel: w467 -> [w486] mode=indexing
                  tunnel: [w482] -> w463
                  i -> [w485]
                  n149 = call "SET_SUPPLY_CHANNEL.vi"("VISA resource name"=w489, "Voltage Level (0.0 V)"=w488, "Enable (OFF)"=TRUE, "Board address"=u8 0, "NChannels"=u8 4, "Channel (0)"=w485, "error in (no error)"=w483, "Voltage Max (0.0 V)"=w487, "Current Limit (0.00 uA)"=w486) -> ("error out"=w482:errorcluster)  [unwired: 6 in]
                }
              }
              frame 1 {
                w502 = 4 ("length")
                w506 = 4 ("length")
                # "Set V to zero"
                n150 = Array Subset(array=w507, length=w506) -> (w509:dbl[])  [unwired: 1 in]
                n151 = Array Subset(array=w508, length=w506) -> (w512:dbl[])  [unwired: 1 in]
                n152 = Array Subset(array=w508, index=w502) -> (w505:dbl[])  [unwired: 1 in]
                n153 = Array Subset(array=w507, index=w502) -> (w504:dbl[])  [unwired: 1 in]
                n154 = for {
                  tunnel: w510 -> [w530]
                  tunnel: w513 -> [w529]
                  tunnel: w512 -> [w526] mode=indexing
                  tunnel: w509 -> [w525] mode=indexing
                  tunnel: [w524] -> w511
                  i -> [w531]
                  w523 = u8 0 ("Board address")
                  n155 = call "SET_SUPPLY_CHANNEL.vi"("VISA resource name"=w530, "Voltage Level (0.0 V)"=w523, "Enable (OFF)"=TRUE, "Board address"=w523, "NChannels"=u8 4, "Channel (0)"=w531, "error in (no error)"=w529, "Voltage Max (0.0 V)"=w526, "Current Limit (0.00 uA)"=w525) -> ("error out"=w524:errorcluster)  [unwired: 6 in]
                }
                n156 = for {
                  tunnel: w501 -> [w514]
                  tunnel: w503 -> [w519]
                  tunnel: w505 -> [w518] mode=indexing
                  tunnel: w504 -> [w517] mode=indexing
                  tunnel: [w515] -> w500
                  i -> [w520]
                  w522 = 0 ("length")
                  n157 = call "SET_SUPPLY_CHANNEL.vi"("VISA resource name"=w514, "Voltage Level (0.0 V)"=w522, "Enable (OFF)"=TRUE, "Board address"=w522, "NChannels"=u8 4, "Channel (0)"=w520, "error in (no error)"=w519, "Voltage Max (0.0 V)"=w518, "Current Limit (0.00 uA)"=w517) -> ("error out"=w515:errorcluster)  [unwired: 6 in]
                }
              }
              frame 2 {
                w534 = 4 ("length")
                w538 = 2 ("length")
                w539 = 4 ("length")
                # "CAEN 2: Top gate, Bottom gate"
                # "CAEN 1 values:\nPMT1&2, Anode, Cathode"
                # "Set VMax to zero, \"Kill\""
                n158 = Array Subset(array=w540, length=w539) -> (w542:dbl[])  [unwired: 1 in]
                n159 = Array Subset(array=w541, length=w539) -> (w545:dbl[])  [unwired: 1 in]
                n160 = Array Subset(array=w540, index=w534, length=w538) -> (w536:dbl[])
                n161 = Array Subset(array=w541, index=w534, length=w538) -> (w537:dbl[])
                n162 = for {
                  tunnel: w543 -> [w565]
                  tunnel: w546 -> [w564]
                  tunnel: w545 -> [w561] mode=indexing
                  tunnel: w542 -> [w559] mode=indexing
                  tunnel: [w558] -> w544
                  i -> [w566]
                  n163 = call "SET_SUPPLY_CHANNEL.vi"("VISA resource name"=w565, "Voltage Level (0.0 V)"=w561, "Enable (OFF)"=TRUE, "Board address"=u8 0, "NChannels"=u8 4, "Channel (0)"=w566, "error in (no error)"=w564, "Voltage Max (0.0 V)"=u8 0 ("Board address"), "Current Limit (0.00 uA)"=w559) -> ("error out"=w558:errorcluster)  [unwired: 6 in]
                }
                n164 = for {
                  tunnel: w533 -> [w547]
                  tunnel: w535 -> [w550]
                  tunnel: w537 -> [w553] mode=indexing
                  tunnel: w536 -> [w551] mode=indexing
                  tunnel: [w549] -> w532
                  i -> [w556]
                  n165 = call "SET_SUPPLY_CHANNEL.vi"("VISA resource name"=w547, "Voltage Level (0.0 V)"=w553, "Enable (OFF)"=TRUE, "Board address"=u8 0, "NChannels"=u8 4, "Channel (0)"=w556, "error in (no error)"=w550, "Voltage Max (0.0 V)"=0, "Current Limit (0.00 uA)"=w551) -> ("error out"=w549:errorcluster)  [unwired: 6 in]
                }
              }
              frame 3, Default {
                # "\"Executes\" if none of the three buttons have been clicked"
                # "Do nothing"
              }
            }
            n166 = Bundle("VISA resource name out"=w442, "error out"=w437) -> (w441:T4)  [unwired: 1 in]
            n167 = Bundle("VISA resource name out"=w440, "error out"=w439) -> (w438:T4)  [unwired: 1 in]
            n168 = Index Array(array=w424) -> (element #1=→"CAEN 1.0":dbl, element #2=→"CAEN 1.1":dbl, element #3=→"CAEN 1.2":dbl, element #4=→"CAEN 1.3":dbl, element #5=→"CAEN 2.0":dbl, element #6=→"CAEN 2.1":dbl, element #7=→"CAEN 2.2":dbl, element #8=→"CAEN 2.3":dbl)  [unwired: 8 in]
          }
          frame #3 {
            # "Descr."
            # "Reset anode"
            n169 = Search 1D Array(1D array=w608, element=TRUE) -> (index of element=w599:i32)  [unwired: 1 in]
            n170 = Not Equal?(x=w599, y=-1) -> (x != y?=w604:bool)
            n171 = case shown="True" "Reset anode" {
              tunnel: w607 -> [_ w642]
              tunnel: w606 -> [_ w618]
              tunnel: w605 -> [_ w623]
              tunnel: w604 -> [_ w643]
              tunnel: [w609 w624] -> w601
              tunnel: w597 -> [_ w617]
              frame False {
                # "Anode Reset Routine inactive:\nkeep timers up to date so activating\nroutine will correctly initiate the timers."
                n172 = Get Date/Time In Seconds() -> (seconds since 1Jan1904=w611:timestamp)
                n173 = To Double Precision Float(number=w611) -> (double precision float=w610:dbl)
                n174 = Build Array(w610, w610) -> (w609:dbl[])
              }
              frame True {
                # "Descr."
                # "0: 1st timer reset, 1: both timers reset, else: do nothing"
                # "Timers"
                # "0: Set to zero, 1: set to value, else: do nothing"
                # "Resetting the timers"
                # "Change Anode Voltage"
                # "Current time > total routine time?"
                # "Current time > target autokill time?"
                n175 = Get Date/Time In Seconds() -> (seconds since 1Jan1904=w652:timestamp)
                n176 = Index Array(array=w642, index #1=0 ("index"), index #2=1 ("index")) -> (element #1=w636:dbl, element #2=w638:dbl)
                n177 = To Double Precision Float(number=w652) -> (double precision float=w637:dbl)
                n178 = case shown="\"CAEN 2\"" "CAEN unit selector" {
                  tunnel: w618 -> [w655 _]
                  tunnel: w617 -> [_ w657]
                  tunnel: [w655 w657] -> w616
                  tunnel: [0 4] -> w614
                  frame "CAEN 1", Default {
                  }
                  frame "CAEN 2" {
                  }
                }
                n179 = Multiply(x="Kill every Y minutes", y=60) -> (x*y=w634:i32)
                n180 = Subtract(x=w637, y=w636) -> (x-y=w635:dbl)
                n181 = Subtract(x=w637, y=w638) -> (x-y=w626:dbl)
                n182 = Add(x=w634, y="Keep off for X seconds") -> (x+y=w625:i32)
                n183 = Greater?(x=w635, y=w634) -> (0:w628:bool)
                "Killed" <- w628
                n184 = Greater?(x=w626, y=w625) -> (0:w629:bool)
                "Restarted" <- w629
                n185 = Or(x=w629, y=w643) -> (x .or. y?=w632:bool)
                n186 = Add(x=w614, y="Anode ch.") -> (x+y=w612:i32)
                n187 = Build Array(w628, w629) -> (w645:bool[])
                n188 = Build Array(w628, w632) -> (w633:bool[])
                n189 = Add(x=w612, y=8) -> (x+y=w619:i32)
                n190 = Add(x=w612, y=16) -> (x+y=w620:i32)
                n191 = Unbundle(w616) -> ("VISA resource name out"=w650:refnum<visa-resource-name>, "error out"=w649:errorcluster)
                n192 = Index Array(array=w623, index #1=w612, index #2=w619, index #3=w620) -> (element #1=w648:dbl, element #2=w646:dbl, element #3=w647:dbl)
                n193 = Search 1D Array(1D array=w645, element=TRUE) -> (index of element=w644:i32)  [unwired: 1 in]
                n194 = Search 1D Array(1D array=w633, element=TRUE) -> (index of element=w630:i32)  [unwired: 1 in]
                n195 = case shown="0" w644 {
                  tunnel: w648 -> [_ w682 _]
                  tunnel: w646 -> [w670 w681 _]
                  tunnel: w647 -> [w672 w680 _]
                  tunnel: w650 -> [w677 w685 _]
                  tunnel: w649 -> [w676 w684 _]
                  tunnel: "Anode ch." -> [w668 w678 _]
                  frame 0 {
                    # "Anode Vset to zero"
                    n196 = call "SET_SUPPLY_CHANNEL.vi"("VISA resource name"=w677, "Voltage Level (0.0 V)"=0.0, "Enable (OFF)"=TRUE, "Board address"=u8 0, "NChannels"=u8 4, "Channel (0)"=w668, "error in (no error)"=w676, "Voltage Max (0.0 V)"=w670, "Current Limit (0.00 uA)"=w672) -> ("error out"=w671:errorcluster)  [unwired: 6 in]
                    n197 = call <vilib>:"Simple Error Handler.vi"("error in (no error)"=w671) -> ()  [unwired: 4 in, 5 out]
                  }
                  frame 1 {
                    # "Anode Vset applied"
                    n198 = call "SET_SUPPLY_CHANNEL.vi"("VISA resource name"=w685, "Voltage Level (0.0 V)"=w682, "Enable (OFF)"=TRUE, "Board address"=u8 0, "NChannels"=u8 4, "Channel (0)"=w678, "error in (no error)"=w684, "Voltage Max (0.0 V)"=w681, "Current Limit (0.00 uA)"=w680) -> ("error out"=w679:errorcluster)  [unwired: 6 in]
                    n199 = call <vilib>:"Simple Error Handler.vi"("error in (no error)"=w679) -> ()  [unwired: 4 in, 5 out]
                  }
                  frame 2, Default {
                    # "Do nothing"
                  }
                }
                n200 = case shown="1" w630 {
                  tunnel: [w658 w664 w667] -> w624
                  tunnel: w642 -> [w662 _ w667]
                  frame 0 {
                    # "Only reset 1st timer, so it\ndoesn't stay True and lock-\nout 2nd check"
                    n201 = Get Date/Time In Seconds() -> (seconds since 1Jan1904=w661:timestamp)
                    n202 = Index Array(array=w662, index=1) -> (element=w659:dbl)
                    n203 = To Double Precision Float(number=w661) -> (double precision float=w660:dbl)
                    n204 = Build Array(w660, w659) -> (w658:dbl[])
                  }
                  frame 1 {
                    # "Reset timers if any button is pressed,\nor if the anode ramps up again"
                    n205 = Get Date/Time In Seconds() -> (seconds since 1Jan1904=w666:timestamp)
                    n206 = To Double Precision Float(number=w666) -> (double precision float=w665:dbl)
                    n207 = Build Array(w665, w665) -> (w664:dbl[])
                  }
                  frame 2, Default {
                    # "Time difference grows \nlarger for now"
                  }
                }
              }
            }
            "Anode times" <- w601
            n208 = To Time Stamp(1:w601) -> (0:→"Anode times 2":timestamp[])
            "?" <- "Reset anode"
          }
          frame #4 {
            # "Temp A, Temp B, Heater%"
            # "To indicators on the physical schematic"
            # "Separate latest 9207 readings.\nIndicators go here"
            # "Displays"
            n209 = local read "Flow input #"() -> (w688:i32)
            n210 = Index Array(array=w691) -> ()  [unwired: 8 in, 8 out]
            n211 = Index Array(array=w691, index=w688) -> (element=w692:dbl)
            n212 = call "Average_flow_x_time.vi"("Array of timestamps"=w696, "Previous Flow"=w695, "Latest Flow"=w692) -> ("Volume (SL)"=w698:dbl)  [unwired: 8 in]
            n213 = case shown="False" "Reset?" {
              tunnel: [w701 0.0] -> w697
              tunnel: w694 -> [w701 _]
              frame False {
              }
              frame True {
              }
            }
            n214 = case shown="True" "Pause?" {
              tunnel: w697 -> [w705 w706]
              tunnel: w698 -> [w704 _]
              tunnel: [w703 w706] -> w693
              frame False {
                n215 = Add(x=w704, y=w705) -> (x+y=w703:dbl)
              }
              frame True {
              }
            }
            "Integrated Flow (SL)" <- w693
            n216 = Index Array(array=w689) -> ()  [unwired: 3 in, 3 out]
            n217 = Index Array(array=w690) -> ()  [unwired: 16 in, 16 out]
            "9207 (V; A) Converted" <- w691
            "9216 #1 (°C)" <- w690
            "9216 #2 (°C)" <- w690
          }
          frame #5 {
            w721 = 16 ("index")
            # "Plots 9207 output vs time"
            # "Descr."
            # "Moving averages"
            # "Historic graphs: Phase, 9207 ai, Flow, Heater, Temperature"
            # "Non-historic Temperature + Det. Pressure"
            # "Updated TOBA"
            # "Descr."
            # "Latest Detector Pressure"
            # "Plots individual lists of Temp. vs. t"
            # "Plots and moving averages"
            n218 = Build Array (concatenate)(w732, w741, w739) -> (w740:dbl[])
            n219 = Build Array (concatenate)(w742, w740) -> (w718:dbl[][])
            "TOBA appended" <- w718
            n220 = local read "Det. T."() -> (w711:i32[])
            n221 = local read "Flow input #"() -> (w707:i32)
            n222 = local read "Det.P input #"() -> (w708:i32)
            n223 = Equal?(x=666, y="Temperature channel selector") -> (x = y?=w733:bool)
            n224 = Index Array(array=w718, index (col)=34 ("disabled index (col)")) -> (element=w726:dbl[])  [unwired: 1 in]
            n225 = case shown="True" w733 {
              tunnel: w732 -> [w787 w793]
              tunnel: w711 -> [_ w792]
              tunnel: [w786 w788] -> w730
              tunnel: "Temperature channel selector" -> [w785 _]
              frame False {
                n226 = Index Array(array=w787, index=w785) -> (element=w786:dbl)
              }
              frame True {
                n227 = for {
                  tunnel: w793 -> [w796]
                  tunnel: w792 -> [w795] mode=indexing
                  tunnel: [w794] -> w789 mode=indexing
                  n228 = Index Array(array=w796, index=w795) -> (element=w794:dbl)
                }
                n229 = Array Size(array=w789) -> (size(s)=w791:i32)
                n230 = Add Array Elements(numeric array=w789) -> (sum=w790:dbl)
                n231 = Divide(x=w790, y=w791) -> (x/y=w788:dbl)
              }
            }
            n232 = Add(x=w708, y=w721) -> (x+y=w723:i32)
            n233 = Add(x=w721, y=w707) -> (x+y=w720:i32)
            n234 = Index Array(array=w718, index (col) #1=w723, index (col) #2=w720) -> (element #1=w722:dbl[], element #2=w719:dbl[])  [unwired: 2 in]
            n235 = Index Array(array=w718, index (col)="Temperature Channel Selector") -> (element=w728:dbl[])  [unwired: 1 in]
            n236 = local read "Det.P input #"() -> (w709:i32)
            n237 = Bundle(w728, w722) -> (w760:cluster{dbl[], dbl[]})  [unwired: 1 in]
            n238 = for {
              N: 8 -> [_]
              tunnel: w718 -> [w777]
              tunnel: w716 -> [w769]
              tunnel: [w774] -> w715 mode=indexing
              tunnel: [w768] -> w714 mode=indexing
              i -> [w773]
              n239 = Add(x=w773, y=24) -> (x+y=w771:i32)
              n240 = Add(x=16, y=w773) -> (x+y=w776:i32)
              n241 = Index Array(array=w777, index (col) #1=w776, index (col) #2=w771) -> (element #1=w775:dbl[], element #2=w770:dbl[])  [unwired: 2 in]
              n242 = Bundle(w769, w775) -> (w774:cluster{timestamp[], dbl[]})  [unwired: 1 in]
              n243 = Bundle(w769, w770) -> (w768:cluster{timestamp[], dbl[]})  [unwired: 1 in]
            }
            "9207 (ai0:7, Volts)" <- w715
            "9207 (ai8:15, Amperes)" <- w714
            n244 = Bundle(w716, w719) -> (w758:cluster{timestamp[], dbl[]})  [unwired: 1 in]
            n245 = Build Array(w758) -> (→"Flow (SLPM)":cluster{timestamp[], dbl[]}[])
            n246 = Index Array(array=w741, index=w709) -> (element=w761:dbl)
            n247 = Build Array(w760) -> (→"Historical Large Phase Diagram":cluster{dbl[], dbl[]}[])
            n248 = Bundle(w730, w761) -> (w765:cluster{dbl, dbl})  [unwired: 1 in]
            n249 = Bundle(w716, w726) -> (w756:cluster{timestamp[], dbl[]})  [unwired: 1 in]
            n250 = Build Array(w756) -> (→"Heater power (%)":cluster{timestamp[], dbl[]}[])
            n251 = Build Array(w765) -> (→"Phase Diagram":cluster{dbl, dbl}[])
            n252 = Reverse 1D Array(array=w722) -> (reversed array=w755:dbl[])
            n253 = Array Subset(array=w755, length="N samples") -> (w745:dbl[])  [unwired: 1 in]
            n254 = Array Size(array=w745) -> (size(s)=w744:i32)
            n255 = local read "Det. T."() -> (w710:i32[])
            n256 = Add Array Elements(numeric array=w745) -> (sum=w754:dbl)
            n257 = Divide(x=w754, y=w744) -> (x/y=→"Detector Pressure":dbl)
            n258 = Equal?(x=666, y="Temperature Channel Selector") -> (x = y?=w735:bool)
            n259 = for {
              N: 16 -> [_]
              tunnel: w716 -> [w813]
              tunnel: [w812] -> w766 mode=indexing
              tunnel: w718 -> [w811]
              i -> [w810]
              n260 = Index Array(array=w811, index (col)=w810) -> (element=w809:dbl[])  [unwired: 1 in]
              n261 = Bundle(w813, w809) -> (w812:cluster{timestamp[], dbl[]})  [unwired: 1 in]
            }
            "Temperature" <- w766
            n262 = case shown="True" w735 {
              tunnel: w732 -> [w799 w805]
              tunnel: w710 -> [_ w804]
              tunnel: [w798 w800] -> w738
              tunnel: "Temperature Channel Selector" -> [w797 _]
              frame False {
                n263 = Index Array(array=w799, index=w797) -> (element=w798:dbl)
              }
              frame True {
                n264 = for {
                  tunnel: w805 -> [w808]
                  tunnel: w804 -> [w807] mode=indexing
                  tunnel: [w806] -> w801 mode=indexing
                  n265 = Index Array(array=w808, index=w807) -> (element=w806:dbl)
                }
                n266 = Array Size(array=w801) -> (size(s)=w803:i32)
                n267 = Add Array Elements(numeric array=w801) -> (sum=w802:dbl)
                n268 = Divide(x=w802, y=w803) -> (x/y=w800:dbl)
              }
            }
            n269 = local read "Channel Names (9207, ai8:15)"() -> (w713:string[])
            n270 = local read "Channel Names (9207, ai0:7)"() -> (w712:string[])
            n271 = Reverse 1D Array(array=w719) -> (reversed array=w751:dbl[])
            n272 = Array Subset(array=w751, length="N samples") -> (w747:dbl[])  [unwired: 1 in]
            n273 = Array Size(array=w747) -> (size(s)=w746:i32)
            n274 = call "Is Value Changed.vim"("value"=w713) -> ("changed or first call?"=w724:bool)
            n275 = call "Is Value Changed.vim"("value"=w712) -> ("changed or first call?"=w725:bool)
            n276 = Add Array Elements(numeric array=w747) -> (sum=w750:dbl)
            n277 = Bundle(w738, w761) -> (w763:cluster{dbl, dbl})  [unwired: 1 in]
            n278 = case shown="True" w724 {
              tunnel: w713 -> [_ w779]
              frame False {
              }
              frame True {
                n279 = for {
                  tunnel: w779 -> [w780] mode=indexing
                  i -> [w781]
                  n280 = property on="9207 (ai8:15, Amperes)" class="XYGraph (strict)"("Active Plot"=w781, "Plot.Plot Name"=w780) -> ()  [unwired: 2 in, 2 out]
                }
              }
            }
            n281 = case shown="True" w725 {
              tunnel: w712 -> [_ w782]
              frame False {
              }
              frame True {
                n282 = for {
                  tunnel: w782 -> [w783] mode=indexing
                  i -> [w784]
                  n283 = property on="9207 (ai0:7, Volts)" class="XYGraph (strict)"("Active Plot"=w784, "Plot.Plot Name"=w783) -> ()  [unwired: 2 in, 2 out]
                }
              }
            }
            n284 = Divide(x=w750, y=w746) -> (x/y=→"Average Flow (SLPM)":dbl)
            n285 = Build Array(w763) -> (→"Large Phase Diagram":cluster{dbl, dbl}[])
          }
          frame #6 {
            # "-----------DATA SAVED----------\nHuman-readable timestamp  ;\nTemperatures (16),  2xNI 9216;\nVolts, Amps  (16),       NI 9207;\nTemperature (2),    Lakeshore;\nHeater power (1),  Lakeshore;\nSetpoint (1),           Lakeshore;\nHV readouts (16)          CAEN ;\nCurrent time (s)                ---   ;\nCycle time (s)                    ---   ;"
            # "Saving data"
            n286 = Get Date/Time In Seconds() -> (seconds since 1Jan1904=w830:timestamp)
            n287 = To Double Precision Float(number=w830) -> (double precision float=w815:dbl)
            n288 = Build Array (concatenate)(w819, w818, w817, w831, w816, w815, w814) -> (w829:dbl[])
            n289 = Get Date/Time String() -> (date string=w823:string)  [unwired: 3 in, 1 out]
            n290 = Build Path(base path=path "D:/Log_data/SC_LOG", name or relative path=w823) -> (appended path=w822:path)
            n291 = Format Date/Time String() -> (date/time string=w827:string)  [unwired: 3 in]
            n292 = Array To Spreadsheet String(array=w829, 3:"%.3f" ("format string")) -> (spreadsheet string=w825:string)  [unwired: 1 in]
            n293 = Concatenate Strings(w827, "\t", w825) -> (w821:string)
            n294 = call <vilib>:"Write Spreadsheet String.vi"("append to file? (new file:F)"=TRUE, "spreadsheet string"=w821, "file path (dialog if empty)"=w822) -> ()  [unwired: 7 in, 2 out]
          }
          frame #7 {
            # "Status is True if any armed\ncondition is met"
            # "Detector P. Alert"
            # "Uninteruptable\n Power Supply Alert"
            # "Temp. Warning"
            # "Arms"
            # "Comm. Alert"
            # "Temperature Alert"
            # "Alarm conditions (Temp)"
            # "Check alarms and UPS"
            n295 = Unbundle By Name(w878) -> ("error out.status"=w856:bool)
            "NI mod 2&3 status" <- w856
            n296 = Unbundle By Name(w891) -> ("error out.status"=w889:bool)
            "LakeShore status" <- w889
            n297 = Unbundle By Name(w893) -> ("error out.status"=w888:bool)
            "CAEN 1 status" <- w888
            n298 = Unbundle By Name(w892) -> ("error out.status"=w887:bool)
            "CAEN 2 status" <- w887
            n299 = Unbundle By Name(w890) -> ("error out.status"=w886:bool)
            "NI mod1 (P) status" <- w886
            n300 = Build Array(w889, w888, w887, w886, w856) -> (w857:bool[])
            n301 = Build Array("LakeShore", "CAEN 1", "CAEN 2", "NI mod 2&3", "NI mod 1") -> (w852:bool[])
            n302 = property on="Det.P input #" class="DigNum (strict)"() -> ("Value"=w872:i32)  [unwired: 2 in, 2 out]
            n303 = Or Array Elements(Boolean array=w857) -> (logical OR=→"Comm. status":bool)
            n304 = for {
              tunnel: w857 -> [w896] mode=indexing
              tunnel: w852 -> [w895] mode=indexing
              tunnel: [w894] -> w851 mode=indexing
              n305 = And(x=w896, y=w895) -> (x .and. y?=w894:bool)
            }
            n306 = Index Array(array=w873, index=w872) -> (element=w869:dbl)
            n307 = Less?(x=w869, y="Underpressure threshold") -> (x < y?=w867:bool)
            n308 = Or Array Elements(Boolean array=w851) -> (logical OR=w841:bool)
            n309 = Greater?(x=w869, y="Overpressure threshold") -> (0:w868:bool)
            n310 = Or(x=w868, y=w867) -> (x .or. y?=w866:bool)
            "Det. P. warning" <- w866
            n311 = And(x=w866, y="Detector P") -> (x .and. y?=w842:bool)
            n312 = call "check_ups.vi"() -> ("Error: no voltages read"=w836:bool, "Timestamp last measured"=→"Timestamp last measured":timestamp, "Minimum input voltage measured"=w846:dbl)  [unwired: 8 in, 1 out]
            "Minimum input voltage measured" <- w846
            n313 = Less?(x=w846, y="UPS Voltage Threshold") -> (x < y?=w838:bool)
            n314 = Equal?(x=w846, y=-1.0) -> (x = y?=w837:bool)
            n315 = local read "Det. T."() -> (w832:i32[])
            n316 = Build Array(w838, w837, w836) -> (w835:bool[])
            n317 = Or Array Elements(Boolean array=w835) -> (logical OR=w834:bool)
            "Warning" <- w834
            n318 = And(x="UPS", y=w834) -> (x .and. y?=w840:bool)
            n319 = Array Size(array=w832) -> (size(s)=w875:i32)
            n320 = Build Array("T 1", "T 2", "T 3", "T 4", "T 5", "T 6") -> (w876:bool[])
            n321 = Array Subset(array=w876, length=w875) -> (w874:bool[])  [unwired: 1 in]
            n322 = for {
              tunnel: w877 -> [w906]
              tunnel: w832 -> [w905] mode=indexing
              tunnel: w874 -> [w899] mode=indexing
              tunnel: [w898] -> w843 mode=indexing
              tunnel: [w897] -> w858 mode=indexing
              n323 = Index Array(array=w906, index=w905) -> (element=w902:dbl)
              n324 = Less?(x=w902, y="Low Temp threshold") -> (x < y?=w901:bool)
              n325 = Greater?(x=w902, y="High Temp threshold") -> (0:w900:bool)
              n326 = Or(x=w901, y=w900) -> (x .or. y?=w897:bool)
              n327 = And(x=w899, y=w897) -> (x .and. y?=w898:bool)
            }
            n328 = Index Array(array=w858) -> (element #1=→"Boolean":bool, element #2=→"Boolean 2":bool, element #3=→"Boolean 3":bool, element #4=→"Boolean 4":bool, element #5=→"Boolean 5":bool, element #6=→"Boolean 6":bool)  [unwired: 6 in]
            n329 = Build Array (concatenate)(w843, w842, w841, w840) -> (w839:bool[])
            n330 = Or Array Elements(Boolean array=w839) -> (logical OR=w833:bool)
          }
          frame #8 {
            # "Testing alarm does not interfere"
            # "Act on alarm"
            n331 = Or(x="Test alarm", y=w912) -> (x .or. y?=w913:bool)
            n332 = case shown="True" w913 {
              tunnel: "Test alarm" -> [_ w917]
              tunnel: w910 -> [_ w931]
              tunnel: w909 -> [_ w929]
              tunnel: w908 -> [w916 w920]
              tunnel: [w916 _] -> w907
              frame False {
                # "Works fine assuming alarm will not need\nto be activated in the first two minutes\nafter the program is ran"
                # "Timer stays at previous value"
              }
              frame True {
                (unwired) "\r\n"
                (unwired) "Temperatures: "
                # "Time to send new SMS"
                # "Average T in Det."
                n333 = Get Date/Time In Seconds() -> (seconds since 1Jan1904=w924:timestamp)
                n334 = To Double Precision Float(number=w924) -> (double precision float=w921:dbl)
                n335 = Multiply(x="Repeat Alarm SMS\nevery N minutes", y=60.0) -> (x*y=w918:dbl)
                n336 = Subtract(x=w921, y=w920) -> (x-y=w919:dbl)
                n337 = case shown="True" w917 {
                  tunnel: ["Error encountered inXAMS! Status:" "TESTING the XAMS alarm. Status:"] -> _
                  frame False {
                  }
                  frame True {
                  }
                }
                n338 = Greater?(x=w919, y=w918) -> ()  [unwired: 1 out]
                n339 = local read "Det.P input #"() -> (w930:i32)
                n340 = Index Array(array=w931, index=w930) -> ()  [unwired: 1 out]
                n341 = local read "Det. T."() -> (w928:i32[])
                n342 = for {
                  tunnel: w929 -> [w944]
                  tunnel: w928 -> [w940] mode=indexing
                  tunnel: [w943] -> w927 mode=indexing
                  tunnel: [w941] -> _ mode=indexing
                  n343 = Format Into String(format string="%.3f", w940) -> (resulting string=w937:string)  [unwired: 2 in, 1 out]
                  n344 = Index Array(array=w944, index=w940) -> (element=w943:dbl)
                  n345 = Format Into String(format string="%.3f", w943) -> (resulting string=w935:string)  [unwired: 2 in, 1 out]
                  n346 = Concatenate Strings("Ch.: " ("format string"), w937, ", Temp.: " ("format string"), w935, ". " ("format string")) -> (w941:string)
                }
                n347 = Array Size(array=w927) -> (size(s)=w925:i32)
                n348 = Add Array Elements(numeric array=w927) -> (sum=w926:dbl)
                n349 = Divide(x=w926, y=w925) -> ()  [unwired: 1 out]
                n350 = Concatenate Strings() -> ()  [unwired: 5 in, 1 out]
              }
            }
            n351 = And(x="Shut off heating if Alarm is active", y=w912) -> (x .and. y?=w914:bool)
          }
        }
        n352 = Decrement(x="Cycles to execute") -> (x-1=w244:dbl)
        n353 = Decrement(x=w244) -> (x-1=w243:dbl)
        n354 = Greater?(x=w227, y=w243) -> ()  [unwired: 1 out]
        n355 = Decrement(x="Clear data every N cycles") -> (x-1=w224:dbl)
        n356 = Greater?(x=w227, y=w224) -> (0:w226:bool)
        n357 = And(x="Auto-clear data?", y=w226) -> (x .and. y?=w229:bool)
        n358 = Or(x=w229, y="Clear data") -> (x .or. y?=w231:bool)
        n359 = case shown="True" w231 {
          tunnel: w242 -> [w272 _]
          tunnel: [w272 dbl[][] []] -> w241
          tunnel: w240 -> [w271 _]
          tunnel: [w271 w278] -> w239
          tunnel: w238 -> [w270 _]
          tunnel: [w270 w278] -> w237
          tunnel: w236 -> [w269 _]
          tunnel: [w269 w276] -> w235
          tunnel: w234 -> [w268 _]
          tunnel: [w268 w274] -> w233
          tunnel: w227 -> [w267 _]
          tunnel: [w267 0] -> w228
          frame False {
          }
          frame True {
            w278 = 0.0
            n360 = Get Date/Time In Seconds() -> (seconds since 1Jan1904=w275:timestamp)
            n361 = To Double Precision Float(number=w275) -> (double precision float=w277:dbl)
            n362 = Build Array(w275) -> (w274:timestamp[])
            n363 = Build Array(w277, w277) -> (w276:dbl[])
          }
        }
        n364 = Or(x=FALSE, y="stop") -> (x .or. y?=w264:bool)
        "Auto-clear" <- "Auto-clear data?"
      }
    }
    frame True {
    }
  }
  n365 = flat-sequence {
    tunnel: w15 -> [w980]
    tunnel: w11 -> [w971]
    tunnel: w10 -> [w968]
    tunnel: w9 -> [w963]
    tunnel: w2 -> [w952]
    frame #0 {
      w976 = u16 2 items=["1"=1, "2"=2] ("Heater Output (1:1)")
      w977 = u16 0 items=["Off", "Low (On)", "Medium", "High"] ("Range (0:Off)")
      # "Turn off heater, shutdown COM"
      # "Error Handling and Post-Processing (EHaPP)"
      n366 = Unbundle(w980) -> ("VISA resource name out"=w979:refnum<visa-resource-name>, "error out"=w978:errorcluster)
      n367 = Unbundle(w971) -> ("VISA resource name out"=w970:refnum<visa-resource-name>, "error out"=w969:errorcluster)
      n368 = Unbundle(w968) -> ("VISA resource name out"=w967:refnum<visa-resource-name>, "error out"=w966:errorcluster)
      n369 = Unbundle(w963) -> ("task out"=w961:refnum<k21>, "error out"=w959:errorcluster)
      n370 = Unbundle(w952) -> ("task out"=w956:refnum<k21>, "error out"=w954:errorcluster)
      n371 = call <vilib>:"DAQmx Stop Task.vi"("task/channels in"=w961, "error in"=w959) -> ("task out"=w960:refnum<k21>, "error out"=w958:errorcluster)  [unwired: 12 in]
      n372 = call <vilib>:"DAQmx Stop Task.vi"("task/channels in"=w956, "error in"=w954) -> ("task out"=w955:refnum<k21>, "error out"=w953:errorcluster)  [unwired: 12 in]
      n373 = call <instrlib>:"Configure Output Range and Manual Value.vi"("VISA resource name"=w979, "Heater Output (1:1)"=w976, "Range (0:Off)"=w977, "Manual Output (0.00 %)"=0.0, "error in (no error)"=w978) -> ("VISA resource name out"=w974:refnum<visa-resource-name>, "error out"=w973:errorcluster)  [unwired: 9 in]
      n374 = call <instrlib>:"Close.vi"("error in (no error)"=w969, "VISA resource name"=w970) -> ("error out"=w965:errorcluster)  [unwired: 9 in]
      n375 = call <instrlib>:"Close.vi"("error in (no error)"=w966, "VISA resource name"=w967) -> ("error out"=w964:errorcluster)  [unwired: 9 in]
      n376 = call <instrlib>:"Close.vi"("error in (no error)"=w973, "VISA resource name"=w974) -> ("error out"=w972:errorcluster)  [unwired: 9 in]
      n377 = call <vilib>:"DAQmx Clear Task.vi"("task in"=w960, "error in"=w958) -> ("error out"=w962:errorcluster)  [unwired: 13 in]
      n378 = call <vilib>:"DAQmx Clear Task.vi"("task in"=w955, "error in"=w953) -> ("error out"=w957:errorcluster)  [unwired: 13 in]
      n379 = call <vilib>:"Simple Error Handler.vi"("error in (no error)"=w972) -> ()  [unwired: 4 in, 5 out]
      n380 = call <vilib>:"Simple Error Handler.vi"("error in (no error)"=w965) -> ()  [unwired: 4 in, 5 out]
      n381 = call <vilib>:"Simple Error Handler.vi"("error in (no error)"=w964) -> ()  [unwired: 4 in, 5 out]
      n382 = call <vilib>:"Simple Error Handler.vi"("error in (no error)"=w962) -> ()  [unwired: 4 in, 5 out]
      n383 = call <vilib>:"Simple Error Handler.vi"("error in (no error)"=w957) -> ()  [unwired: 4 in, 5 out]
    }
  }
  n384 = Array Size(array=w25) -> (size(s)=w28:i32)
  n385 = Decrement(x=w28) -> (x-1=w27:i32)
  n386 = Index Array(array=w25, index #1=w27, index #2=1 ("index")) -> (element #1=w26:timestamp, element #2=w7:timestamp)
  n387 = To Double Precision Float(number=w26) -> (double precision float=w24:dbl)
  n388 = To Double Precision Float(number=w7) -> (double precision float=w23:dbl)
  n389 = Subtract(x=w24, y=w23) -> ()  [unwired: 1 out]
  "Started up?" <- w19
